vi "MultiClassTable.vi"() -> ()   [LabVIEW 2013]
uses:
  ColumnVIs/Column/Column.lvclass
  ColumnVIs/ModeCol/ModeCol.lvclass
  ColumnVIs/GroupCol/GroupCol.lvclass
  ColumnVIs/DigitalCol/DigitalCol.lvclass
  ColumnVIs/TriggerCol/TriggerCol.lvclass
  ColumnVIs/SingleValCol/SingleValCol.lvclass
  <vilib>/event_ctls.llb/eventvkey.ctl
  <vilib>/Utility/miscctls.llb/LVRowAndColumnTypeDef.ctl
  TypeDefs/RowType.ctl
  TypeDefs/TableHistory.ctl
  TypeDefs/TableArray.ctl
  TypeDefs/AddDeviceRing.ctl
  DeviceVIs/Device/Device.lvclass
  TypeDefs/PreviousVersionSelect.ctl
  VariableManagerCodes/VariableManager/VariableManager.lvclass
  <vilib>/Utility/miscctls.llb/LVRowAndColumnUnsignedTypeDef.ctl
  PackedLibraries/LuaEvaluatorAPI.lvlibp/API/t_Caching_Expression_Evaluator_Methods_v4.ctl
  TypeDefs/ClickEvent.ctl
  <vilib>/Utility/miscctls.llb/LVPoint32TypeDef.ctl
  <vilib>/Utility/error.llb/DialogType.ctl
  TypeDefs/SaveCluster.ctl
  <vilib>/Utility/miscctls.llb/LVStringsAndValuesArrayTypeDef_I32.ctl
  <vilib>/Utility/cursorutil.llb/Set Cursor (Icon Pict).vi
  DeviceVIs/NextMaster_v4.vi
  PackedLibraries/LuaEvaluatorAPI.lvlibp
  DeviceVIs/SubVIs.lvlib
  VariableManagerCodes/API/VariableManagerAPI.lvlib
panel:
  out "Button\n(Mouse Down?)":u16
  out "Index Values":T1
  out "Igor Inform Array":string[](array[string])
  out "Devices queue":refnum<queue>
  in  "UpdateHWI Button":bool
  in  "StopExperiment":bool
  in  "Run Seq Button":bool
  in  "Run Button":bool
  in  "Cycle":bool
  in  "RandomSequence":bool
  in  "VariableManager":refnum<class "VariableManager.lvclass">=refnum
  out "CycleX Event":refnum<user-event>
  out "Dyn.\nRegist.\nCycleX\nEvent":refnum<event-registration>
  out "Dyn.\nRegist.\nSeq.\nEvent":refnum<event-registration>
  out "Dyn. Regist. Update Event":refnum<event-registration>
  out "Update Notifier":refnum<notifier>
  out "Update Event":refnum<user-event>
  out "Seq. Event":refnum<user-event>
  out "Loaded Version":string="testing"
  out "Procedure Name":string="test_branch"
  in  "Tab Control":T2(tab)=enum."Variables"
  in  "Program only changes":bool=TRUE
  out "SequenceHistory":string[][](table)
  in  "File Number":i32
  in  "Program during MOT loading":bool
  in  "Additional wait time (s)":dbl
  out "Igor Inform String":string
  in  "FitCol2Text Button":bool
  in  "SetList Table":string[][](table)=[["initialize", "", "Ramp", "1", "1", "0", "0", "0", "0", "0", "0", "0", "0", "0", "0", "0", "0", "0", "0", "0", "0", "0", "0", "0", "0", "0", "0", "0", "0", "100m"]]
  in  "Undo":bool
  in  "Redo":bool
  in  "Select Layout":i32(ring)=-1 items=["(On-the-fly)"=-2, "All"=-1]
  in  "ConfigLayoutsButton":bool
  in  "Add Device":T3 items=["Select Type...", "DDS", "Novatech", "NI Card"]
  in  "ManageDevicesButton":bool
  in  "User defined functions":string="-- --------------------------------------------------------------------------\n-- RbYb Beatnote Command \"frequency\" functions\n--      These functions allow us to run a sequence using absolute frequency \n--      detuning by calculating the proper command \"frequency\"\n--\n--      NOTE: Only use one TA or Re \"comm\" function, or it isn't clear which setpoint will be used\n--\n--      18.Aug.2010: Updated Master AOM offset (40 --> 42.342).\n-----------------------------------------------------------------------------\nfunction TASlowComm(Detuning,AOM)\n    return (-1*Detuning+1126.48-60.32-42.342-2*AOM)/8\n   --positive detuning is BLUE detuned, zero detuning sets TA slower beam to the 87-Rb F=2 to F'=3\nend\n\nfunction TAMOTComm(Detuning,AOM)\n    return (-1*Detuning+1126.48-60.32-42.342+AOM)/8\n   --positive detuning is BLUE detuned, zero detuning sets TA MOT beam to the 87-Rb F=2 to F'=3\nend\n\nfunction TAPComm(Detuning,AOM)\n    return (-1*Detuning+1126.48-60.32-42.342+AOM)/8\n   --positive detuning is BLUE detuned, zero detuning sets TA Probe beam to the 87-Rb F=2 to F'=3\nend\n\nfunction ReMOTComm(Detuning,AOM)\n    return (Detuning+6568.03-1126.48+60.32+42.342-2*AOM)/64\n    --positive detuning is BLUE detuned, zero detuning sets Repump MOT beam to the 87-Rb F=1 to F'=2\nend\n\nfunction ReSlowComm(Detuning,AOM)\n    return (Detuning+6568.03-1126.48+60.32+42.342+2*AOM)/64\n    --positive detuning is BLUE detuned, zero detuning sets Repump slower beam to the 87-Rb F=1 to F'=2\nend\n\n--RbLi Probe (transverse coolign launch)\nfunction PComm(Detuning)\n    return (-1*Detuning+986.16)/8\n    --positive detuning is BLUE detuned, zero detuning sets Repump slower beam to the 87-Rb F=1 to F'=2\nend\n\n-- Creates an exponential ramp from A to B in tEnd seconds\n-- useful for stopping a ramp at different times to measure T, N\nfunction ExpRampStep(t, a, b, tau, tEnd)\n   return (b - a*exp(tEnd / tau) + (a-b)*exp(t/tau))/ ( 1 - exp(tEnd / tau) );\nend\n\nfunction ExpRampEnd(tEv, a, b, tau, tEnd)\n   return (b - a*exp(tEnd / tau) + (a-b)*exp(tEv/tau))/ ( 1 - exp(tEnd / tau) );\nend\n\nfunction ExpRamp2(t,a,tau)\n   return a*exp(-t/tau)\nend\n\nfunction ExpRamp2End(tEnd,a,tau)\n   return a*exp(-tEnd/tau)\nend\n\n-- Added log chip amplifier (1 V per decade) so now we provide linear ramp to get exponential\n--     note: log() is base 'e', log10 base '10'\nfunction LineEvap(t,a,tau)\n   return 1.027*(log10(a)-t/(2.30*tau))+0.0343\nend\n\n-- final value log(V) for LineEvap\nfunction LineEvapEnd(tEnd,a,tau)\n   return 1.027*(log10(a)-tEnd/(2.30*tau))+0.0343\nend\n\n-- Convert real dipole power to log chip request V\nfunction PtoV(pow)\n   return 1.010*log10(pow/0.770)\nend\n\n-- Convert 532 horizontal (main) beam power (in mW) to V-req\nfunction PtoV532m(pow)\n   return 1.01378*log10(pow/0.54672)\nend\n\n-- Convert 532 vertical (crossing) beam power (in mW) to V-req\nfunction PtoV532c(pow)\n   return 1.03459*log10(pow/0.619665)\nend\n\n-- Convert 1064 horizontal (main) beam power (in mW) to V-req\nfunction PtoV1064m(pow)\n   return 1.0035*log10(pow/1.2104)\nend\n----------------------------------------\n-- The following functions are part of the \"standard load\" of functions and should not be messed with\n-- They are here for reference only.\n-- Please add any user functions above this comment\n-- -------------------------------------------------------------------------------------------\n\n-- Creates a linear ramp from A to B\nfunction LineRamp(f, Initial, Final)\n    return (1-f)*Initial + f*Final;\nend\n\n-- Creates an exponential ramp from A to B\nfunction ExpRamp(t, a, b, tau)\n   return (b - a*exp(tMax / tau) + (a-b)*exp(t/tau))/ ( 1 - exp(tMax / tau) );\nend\n\n-- Creates a sinewave\nfunction SinRamp(t,Offset,A,Freq, Phase)\n    return Offset + A * sin(2*pi*Freq*t + Phase)\nend\n\n-- Creates a blackman pulse\nfunction Blackman(f, Offset, A)\n    return Offset +  A*sqrt(0.5*cos(3.1415*(2*f-1))+0.08*cos(2*pi*(2*f-1))+0.42);\nend\n\n-- Creates a half-gauss ramp\nfunction HalfGaussRamp(t, a, b, Width)\n    local y;\n    y = exp(-(tMax^2)/Width^2);\n    y = (a -  b*y)/(1-y)  +  ((b-a)/(1-y))*exp(-((t-tMax)^2)/Width^2);\n    return y;\nend\n\n-- Creates an \"O'Hara\" ramp from A to B, for dipole evaporation\nfunction EvapRamp(t, a, b, tau)\n   local y;\n  y = log(a/b) / log(1+tMax/tau);\n  y = a * (1+t/tau)^(-y);\n  return y;\nend\n"
  out "Loading Text":string="Loading..."
  in  "Version Selection":T4=enum."Load DDS 4.10"
  in  "Old HWGlobals Path":path=path "C:/Experiment/Data Acquisition/Hardware Control/Hardware/2014/6Jun2014_PowerCal" caption="This file has not been loaded or saved"
  in  "Old HWGlobals History":string(combo)
  in  "Old Procedure Path":path=path "C:/Experiment/Data Acquisition/Hardware Control/procedures/Benchmarks/12Feb2014_RbQuad" caption="This file has not been loaded or saved"
  in  "Old Procedure History":string(combo)
  in  "Load Old":bool
  in  "Load Recent":string(combo)
  in  "Save to Disk":bool
  in  "Load from Disk":bool
  out "Table error":errorcluster
  out "Sequencing Error":errorcluster
  out "Update Error":errorcluster
  in  "Debug: apply appearance":bool
  out "DevNums":i32[](array[numeric])=[0, 0, 0, 0, 0, 0, 0, 0, 0, 0, 0, 0, 0, 0, 0, 0, 0, 0, 0, 0, 0, 0, 0, 0, 0, 0, 0, 0, 0, 0, 1, 1, 1, 1, 1, 1, 1, 1, 1, 1, 1, 1, 1, 1, 1, 1, 1, 1, 1, 1, 2, 2, 2, 2, 2, 2, 2, 2, 2, 2, 2, 2, 2, 2, 2, 2, 2, 2, 2, 2, 3, 3, 3, 3, 3, 3, 3, 3, 3, 3, 3, 3, 3, 3, 3, 3, 3, 3, 3, 3, 4, 4, 4, 4, 4, 4, 4, 4, 5, 5, 5, 5, 5, 5, 5, 5, 5, 5, 5, 5, 6, 6, 6, 6, 6, 6, 6, 6, 6, 6, 6, 6, 7, 7, 7, 7, 7, 7, 7, 7, 7, 7, 7, 7]
  in  "Devices":refnum<class "Device.lvclass">[](array[class])
  in  "PreserveHist?":bool
  out "Hist. size":i32=2
  out "#chg":i16
  out "Defer Pnl Upd":bool=TRUE
  out "diag. loop cnt":i32
  out "Key Focus":bool
  out "Edit Position":T5={"Row"=-2, "Column"=-2}
  out "withinSelection?":bool
  out "Val Change":bool=TRUE
  out "Selection Size":T5
  in  "row type":T6=enum."within data"
  out "Selection Start":T5={"Row"=25, "Column"=30}
  out "Char":i16
  out "VKey":T7
  out "withinData?":bool=TRUE
  out "data cols":i32=134
  out "data rows":i32=26
  out "Number of Rows":u32=36
  out "Number of Columns":u32=62
  out "Table History":T8
  in  "Diag. loop?":bool
  in  "Defer Updates?":bool=TRUE
  out "Clipboard":string[][](array[string])
  out "Col array":refnum<class "Column.lvclass">[](array[class])
  in  "quit":bool
  in  "initialize?":bool
  # "Use the quit button -->\nPressing stop causes problems with Variable Manager"
  # "(must abort to stop,\nstill better to QUIT first)"
  # "diagnostics:"
  # "presently not set\nfor row header"
  # "The table size in (rows, cols) is NOT same as\nthe size of the data array displayed in table."
  # "Necessary table settings:\n - Show column/row headers (Properties)\n - No editable headers (unless we'll handle all column header clicks)"
  # "\"Diagnostics\" we can't delete:\nRow Type, ..."
  # "What do we actually need from old CycleX here?\n   - Inform Igor?\n   - Program changes/ during MOT load?"
  # "(not presently implemented)"
  # "Sequencing controls to add: Run Sequence/Abort, Sequence Step indicator, Randomize?, Mulligans"
  # "Variable Manager will be initialized when the VI is run.\n\nIf it is currently running and you can see this message, then you've \"popped out\" the Variable manager.\nClose it with the \"red-x\" to replace it here."
  # "Note: For each index <idx>, the names <idx>_f and <idx>_max\nare also defined as the fractional sequence step and max steps."
  # "In the context of ramps several variables are passed or specified that may be used here:\n\n   - f the fractional position of a point in a ramp\n   - t the current time in a ramp\ndt the current timestep size.\ntMax the total duration of the ramp\n\ntemporary \"storage\":\n-- not functionality for strings (always treated as double)\nfunction bnot(a)\n   -- this \"(bool exp.) and b or c\" is equivalent to \"(bool exp.) ? b : c\" syntax.\n   -- caution: undefined variables evaluate to \"false\" so will NOT throw an error as argument\n   return a==0 and 1 or 0\nend"
  # "Present Version"
  # "Save/Load from present version (select single file):\nWe need to save the following:\n   - Devices (with the columns and data pushed from table first!)\n   - Layout ring (for layout names, #s)\n   - variables\n   - user functions\n   - ... ?"
  # "Load... and Save... bring up dialog box.\nLoad Recent will load the selected procedure. BUG: not a value change if select what's on top!"
  # "Previous Versions"
  # "Load from older versions (select Procedure and Hardware globals)\n(1) reformat old file to give device array\n(2) collect variables and send them to variable manager\n(3) load user functions\n(4) construct layouts, if any (at least a default \"all on\" layout)\n(5) ...?"
  # "Notes:\n\nVariables used in digital columns are interpreted as high for any value not equal to 0, and low for 0."
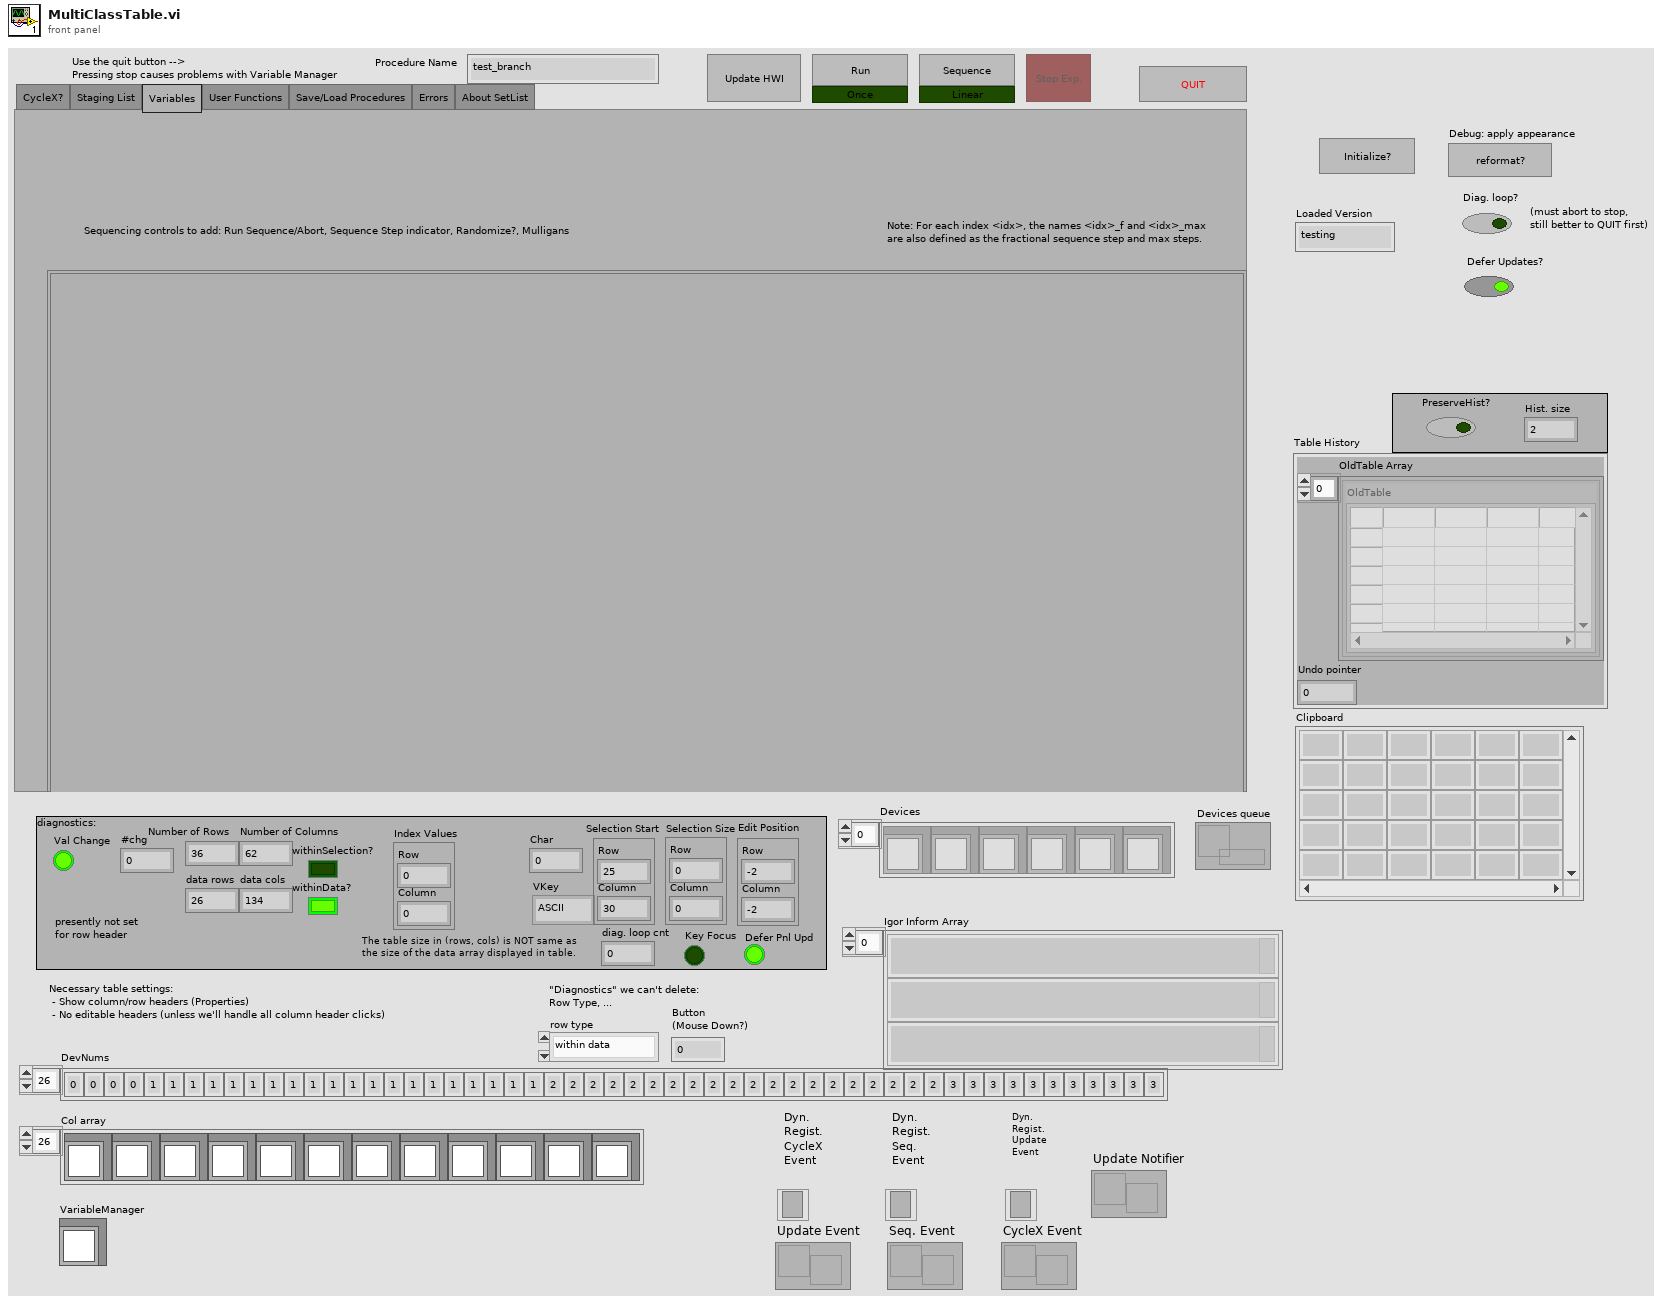
[diagram p1: front panel]
types:
  T1 = typedef "LVRowAndColumnUnsignedTypeDef.ctl" = cluster{"Row":u32, "Column":u32}
  T2 = enum32{"CycleX?", "Staging List", "Variables", "User Functions", "Save/Load Procedures", "Errors", "About SetList"}
  T3 = typedef "AddDeviceRing.ctl" = u16
  T4 = typedef "PreviousVersionSelect.ctl" = enum32{"Load PreDDS 4.10", "Load early 2009 files", "Load 2009-2010 files", "Load DDS 4.10", "Load v4.09"}
  T5 = typedef "LVRowAndColumnTypeDef.ctl" = cluster{"Row":i32, "Column":i32}
  T6 = typedef "RowType.ctl" = enum16{"below data", "within data", "column header", "first row"}
  T7 = typedef "eventvkey.ctl" = enum16{"ASCII", "Enter", "Return", "Shift", "Ctrl", "Alt", "Cmd", "Opt", "Caps", "NumLock", "Clear", "Break", "Up", "Down", "Left", "Right", "Insert", "Delete", "Home", "End", "PageUp", "PageDown", "Escape", "Help", "Pause", "ScrollLock", "F1", "F2", "F3", "F4", "F5", "F6", "F7", "F8", "F9", "F10", "F11", "F12", "F13", "F14", "F15", "F16", "F17", "F18", "F19", "F20", "F21", "F22", "F23", "F24", "Play", "VolumeUp", "VolumeDown", "Mute", "Two Byte Char"}
  T8 = typedef "TableHistory.ctl" = cluster{"OldTable Array":T9, "Undo pointer":i32}
  T9 = typedef "TableArray.ctl" = cluster{"OldTable":string[][]}[]
  T10 = enum8{"Enabled", "Disabled", "Disabled and Grayed Out"}
  T11 = typedef "LuaEvaluatorAPI.lvlibp/t_Caching_Expression_Evaluator_Methods_v4.ctl" = enum16{"set", "get", "eval", "eval2", "assign", "execute", "isvalid"}
  T12 = typedef "ClickEvent.ctl" = cluster{"CtlRef":refnum<vi>, "Coords":T13, "Button":u16, "Mods":cluster{"Double Click":bool, "Menu Key":bool}, "PlatMods":cluster{"Shift":bool, "Ctrl":bool, "Alt":bool, "Cmd":bool, "Opt":bool}}
  T13 = typedef "LVPoint32TypeDef.ctl" = cluster{"Horizontal":i32, "Vertical":i32}
  T14 = typedef "SaveCluster.ctl" = cluster{"Version":string, "Devices":refnum<class "Device.lvclass">[], "Select Layout":i32, "Layout:Strings And Values []":T15, "User defined functions":string, "VariableManager":refnum<class "VariableManager.lvclass">}
  T15 = typedef "LVStringsAndValuesArrayTypeDef_I32.ctl" = cluster{"String":string, "Value":i32}[]
  T16 = cluster{"Shift":bool, "Ctrl":bool, "Alt":bool, "Cmd":bool, "Opt":bool}
  T17 = typedef "ClickReturn.ctl" = cluster{"Button":u16, "Mods":cluster{"Double Click":bool, "Menu Key":bool}, "PlatMods":cluster{"Shift":bool, "Ctrl":bool, "Alt":bool, "Cmd":bool, "Opt":bool}, "Discard?":bool}
  T18 = typedef "DialogType.ctl" = u16
  T19 = typedef "ColumnLayoutCluster.ctl" = cluster{"Label":string, "Color":u32, "Width":u32, "[disp?]":bool[]}
  T20 = cluster{"left":i16, "top":i16, "right":i16, "bottom":i16}
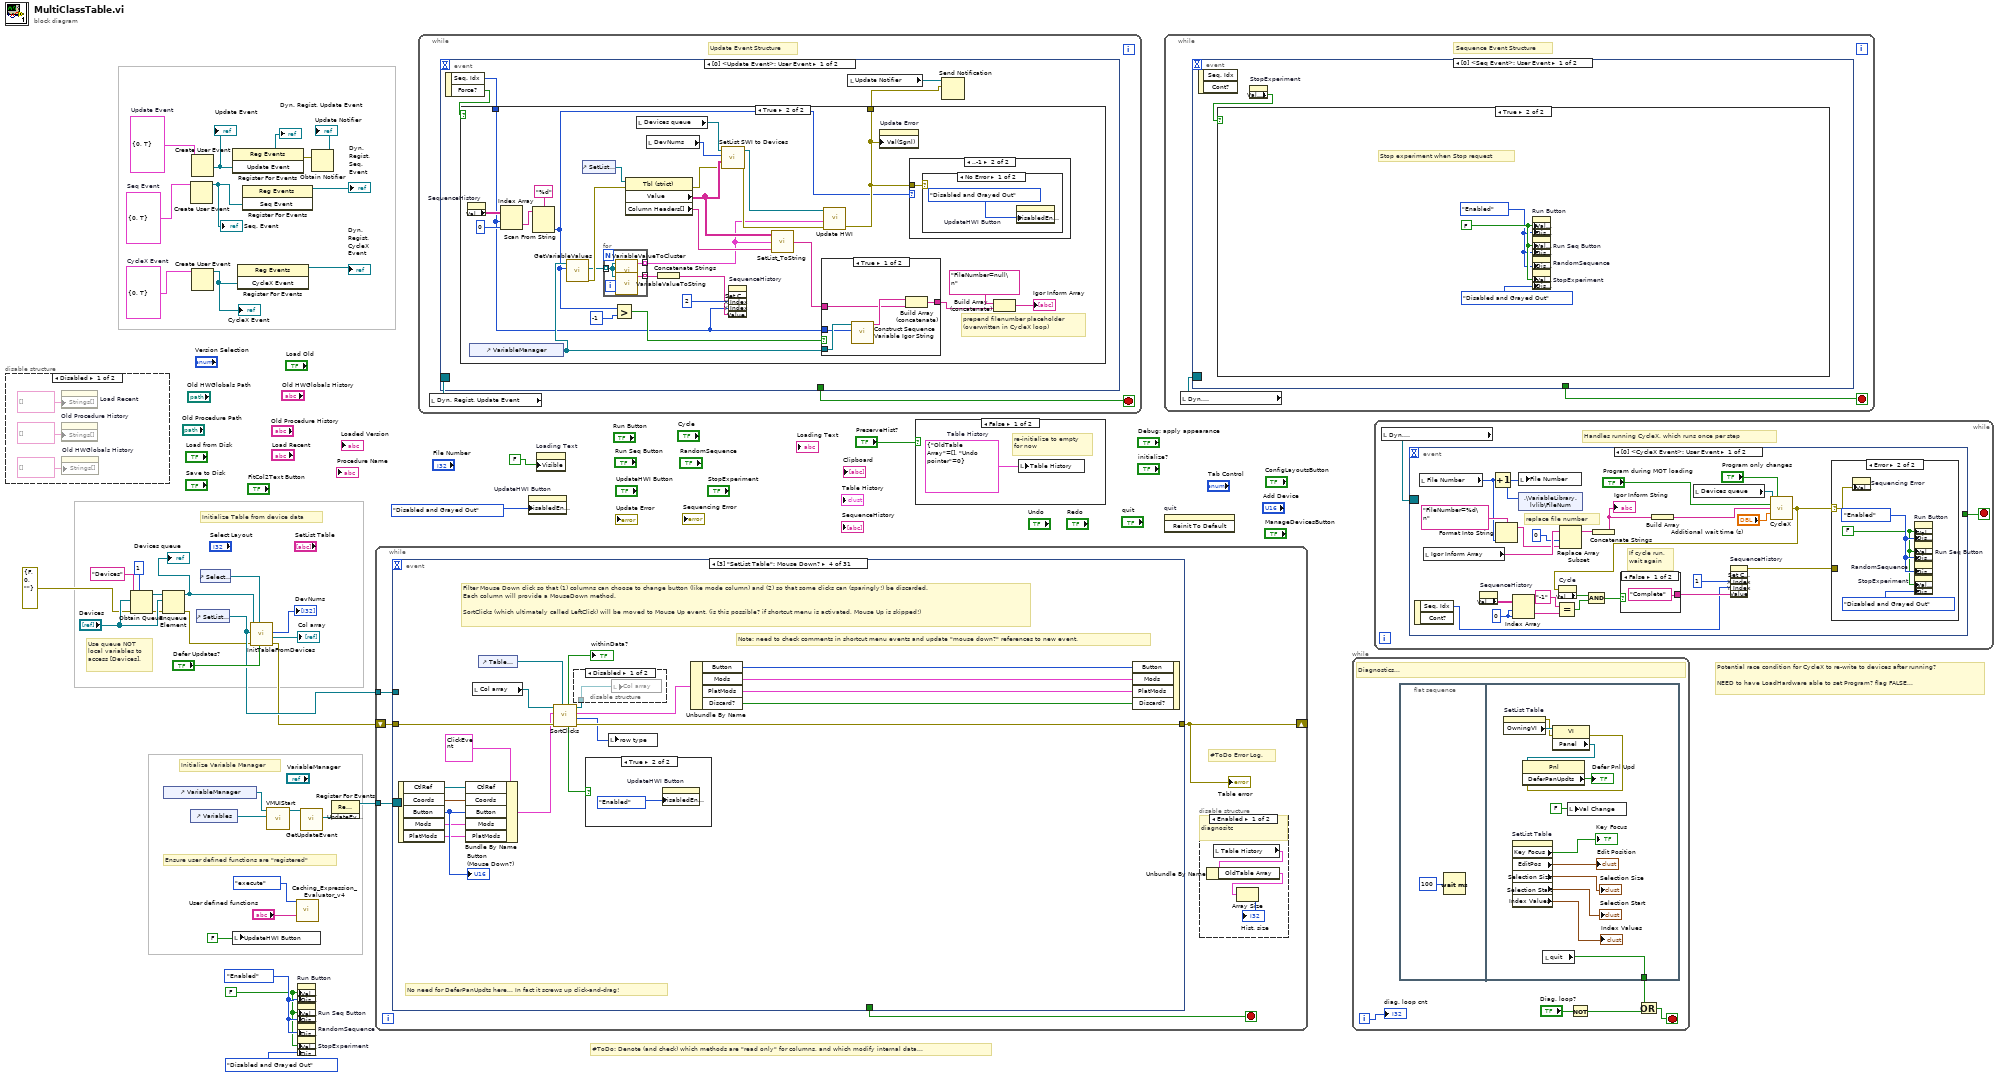
[diagram p0: block diagram]
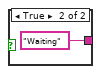
[diagram p2: hidden frame]
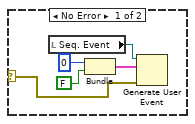
[diagram p3: hidden frame]
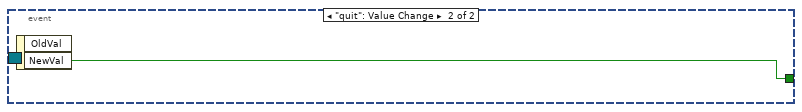
[diagram p4: hidden frame]
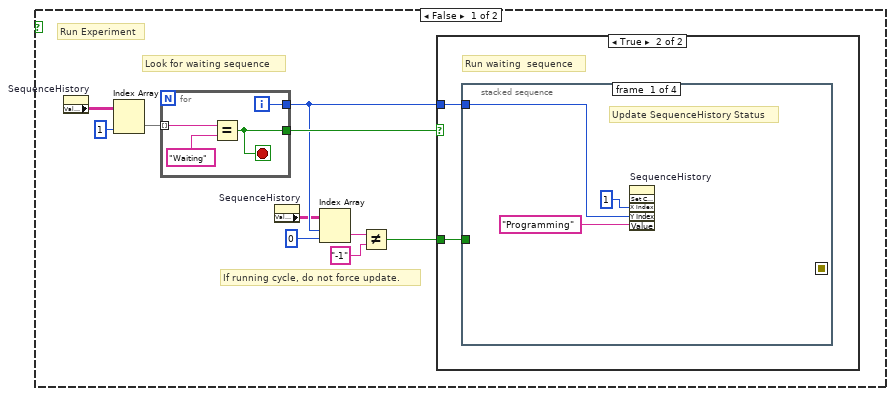
[diagram p6: hidden frame]
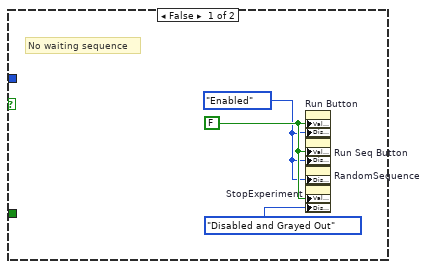
[diagram p7: hidden frame]
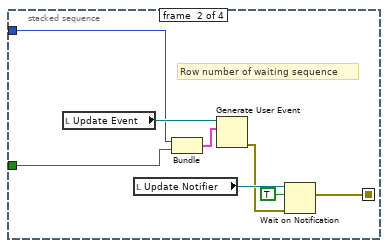
[diagram p8: hidden frame]
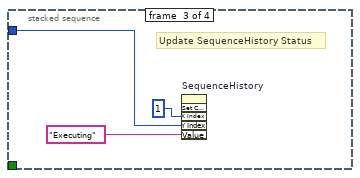
[diagram p9: hidden frame]
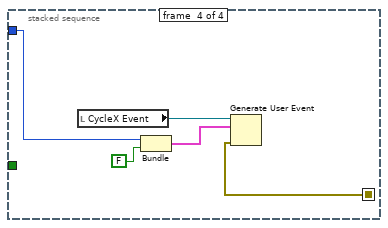
[diagram p10: hidden frame]
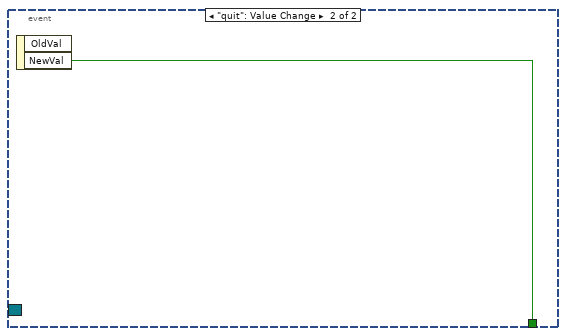
[diagram p11: hidden frame]
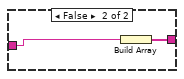
[diagram p15: hidden frame]
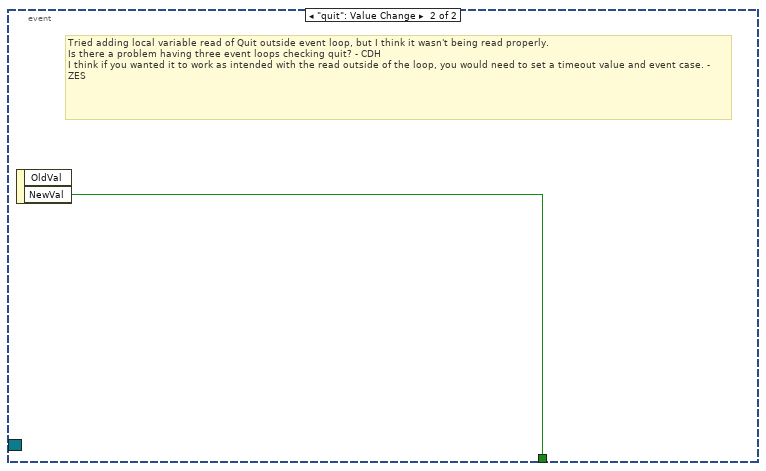
[diagram p16: hidden frame]
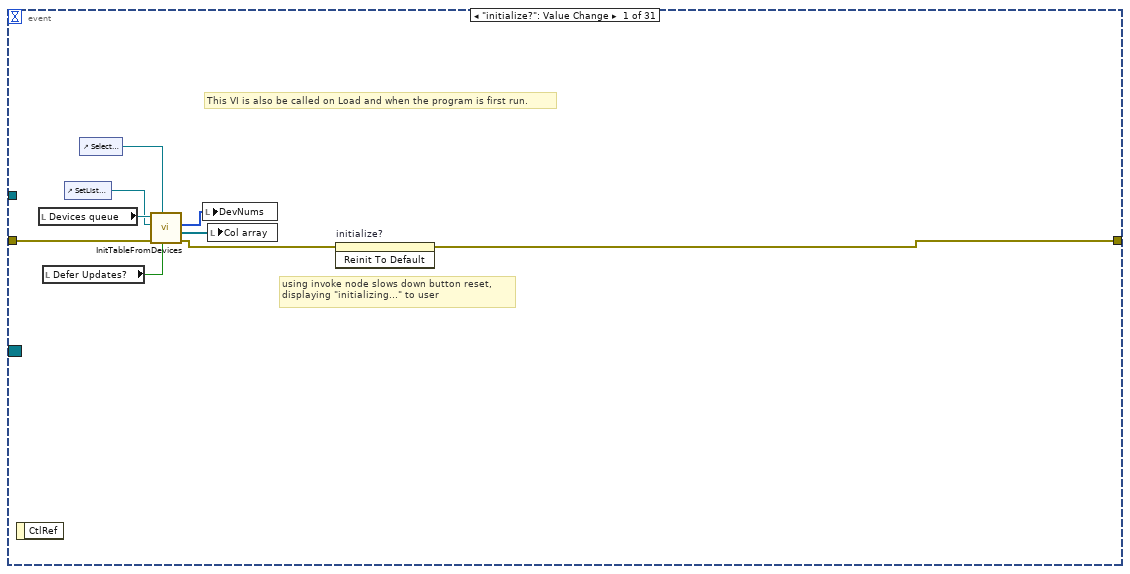
[diagram p19: hidden frame]
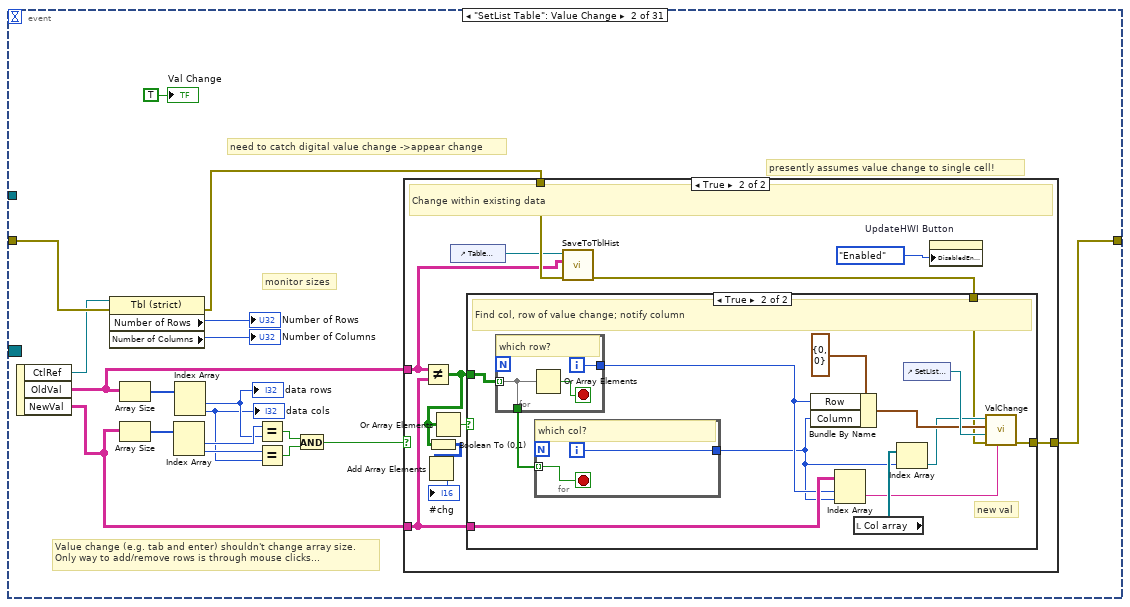
[diagram p20: hidden frame]
diagram:
  w13 = T10."Enabled" ("Disabled")
  w12 = FALSE
  w24 = cluster{"Seq. Idx":i32, "Cont?":bool} {"Seq. Idx"=0, "Cont?"=TRUE}  # CycleX Event
  w36 = cluster{"Seq. Idx":i32, "Cont?":bool} {"Seq. Idx"=0, "Cont?"=TRUE}  # Seq Event
  w37 = cluster{"Seq. Idx":i32, "Force?":bool} {"Seq. Idx"=0, "Force?"=TRUE}  # Update Event
  # "Use queue NOT\nlocal variables to\naccess [Devices]."
  # "Potential race condition for CycleX to re-write to devices after running?\n\nNEED to have LoadHardware able to set Program? flag FALSE..."
  # "Ensure user defined functions are \"registered\""
  # "Initialize Variable Manager"
  # "Initialize Table from device data"
  # "#ToDo: Denote (and check) which methods are \"read only\" for columns, and which modify internal data..."
  n1 = disable-structure shown="Disabled" {
    frame Disabled {
      n2 = property on="Load Recent" class="CmbBox"("Strings[]"=string[] [] ("Strings []")) -> ()  [unwired: 2 in, 2 out]
      n3 = property on="Old Procedure History" class="CmbBox"("Strings[]"=string[] [] ("Strings []")) -> ()  [unwired: 2 in, 2 out]
      n4 = property on="Old HWGlobals History" class="CmbBox"("Strings[]"=string[] [] ("Strings []")) -> ()  [unwired: 2 in, 2 out]
    }
    frame Enabled {
    }
  }
  n5 = Obtain Queue(max queue size (-1, unlimited)=1, name (unnamed)="Devices", element data type="Devices", error in (no error)=errorcluster {"status"=FALSE, "code"=0, "source"=""} ("error out")) -> (queue out=w5:refnum<queue>, error out=w4:errorcluster)  [unwired: 1 in, 1 out]
  n6 = Enqueue Element(queue=w5, element="Devices", error in (no error)=w4) -> (queue out=w1:refnum<queue>, error out=w3:errorcluster)  [unwired: 1 in, 1 out]
  "Devices queue" <- w1
  n7 = control-ref of="VariableManager"() -> (w16:refnum<vi>)
  n8 = control-ref of="Variables"() -> (w15:refnum<vi>)
  n9 = Create User Event(user event datatype=w36) -> (user event=w21:refnum<user-event>)  [unwired: 1 in, 1 out]
  "Seq. Event" <- w21
  n10 = Create User Event(user event datatype=w37) -> (user event=w38:refnum<user-event>)  [unwired: 1 in, 1 out]
  "Update Event" <- w38
  n11 = Create User Event(user event datatype=w24) -> (user event=w23:refnum<user-event>)  [unwired: 1 in, 1 out]
  "CycleX Event" <- w23
  n12 = control-ref of="SetList Table"() -> (w18:refnum<vi>)
  n13 = control-ref of="Select Layout"() -> (w30:refnum<vi>)
  n14 = register-events(w38) -> (reference out=→"Dyn. Regist. Update Event":refnum<event-registration>, error out=w32:errorcluster)  [unwired: 2 in]
  n15 = local write "UpdateHWI Button"(FALSE ("UpdateHWI Button")) -> ()
  n16 = register-events(w23) -> (reference out=→"Dyn.\nRegist.\nCycleX\nEvent":refnum<event-registration>)  [unwired: 2 in, 1 out]
  n17 = register-events(w21) -> (reference out=→"Dyn.\nRegist.\nSeq.\nEvent":refnum<event-registration>)  [unwired: 2 in, 1 out]
  n18 = call "InitTableFromDevices.vi"("Defer Updates? (T)"="Defer Updates?", "Layout Ref"=w30, "error in (no error)"=w3, "Table Ref in"=w18, "Devices queue"=w1) -> ("error out"=w17:errorcluster, "Col array"=→"Col array":refnum<class "Column.lvclass">[], "DevNums"=→"DevNums":i32[])  [unwired: 3 in, 1 out]
  n19 = call "VMUIStart.vi"("SubPanelRef"=w15, "VariableManagerRef in"=w16) -> ("VariableManagerRef out"=w11:refnum<vi>)  [unwired: 8 in, 1 out]
  n20 = call "Caching_Expression_Evaluator_v4.vi"("method"=t_Caching_Expression_Evaluator_Methods_v4."execute", "expression/scriptlet"="User defined functions") -> ()  [unwired: 12 in, 2 out]
  n21 = property on="Run Button" class="Bool (strict)"("Value"=w12, "DisabledEnum"=w13) -> ()  [unwired: 2 in, 2 out]
  n22 = property on="Run Seq Button" class="Bool (strict)"("Value"=w12, "DisabledEnum"=w13) -> ()  [unwired: 2 in, 2 out]
  n23 = property on="RandomSequence" class="Bool (strict)"("DisabledEnum"=w13) -> ()  [unwired: 2 in, 2 out]
  n24 = property on="StopExperiment" class="Bool (strict)"("Value"=w12, "DisabledEnum"=T10."Disabled and Grayed Out" ("Disabled")) -> ()  [unwired: 2 in, 2 out]
  n25 = call "GetUpdateEvent.vi"("VariableManagerRef in"=w11) -> ("UpdateEvent"=w10:refnum<user-event>)  [unwired: 8 in, 2 out]
  n26 = Obtain Notifier(notification data type=w32) -> (notifier out=→"Update Notifier":refnum<notifier>)  [unwired: 3 in, 2 out]
  n27 = register-events(w10) -> (reference out=w9:refnum<event-registration>)  [unwired: 2 in, 1 out]
  n28 = while {
    shift-right: [w45] -> _
    shift-left: w17 -> [w46]
    tunnel: w18 -> [w44]
    tunnel: w9 -> [w43]
    stop <- w47 stop-if-true
    # "#ToDo Error Log."
    n29 = event shown="[3] \"SetList Table\": Mouse Down?" {
      selector: w43 -> [_ _ _ _ _ _ _ _ _ _ _ _ _ _ _ _ _ _ _ _ _ _ _ _ _ _ _ _ _ _ _]
      dyn-events: _ -> [_ _ _ _ _ _ _ _ _ _ _ _ _ _ _ _ _ _ _ _ _ _ _ _ _ _ _ _ _ _ _]
      timeout: _ -> [_ _ _ _ _ _ _ _ _ _ _ _ _ _ _ _ _ _ _ _ _ _ _ _ _ _ _ _ _ _ _]
      tunnel: [_ _ _ _ _ _ _ _ _ _ _ _ _ _ _ w477 _ _ _ _ _ _ _ _ _ _ _ _ _ _ _] -> w47
      tunnel: [w51 w61 w115 w215 _ w281 w298 w316 w319 w324 w341 w350 w365 w431 _ w468 w484 w510 _ _ _ _ _ _ w639 _ _ w652 _ _ _] -> w45
      tunnel: w46 -> [w54 w65 w114 w216 w231 w280 w310 w317 w320 w325 w344 w352 w368 w428 _ w471 w482 w512 _ _ _ _ _ _ w635 _ _ _ _ _ _]
      tunnel: w44 -> [_ _ _ _ _ _ _ _ _ _ w340 _ w367 w426 _ _ w480 w507 _ _ _ _ _ _ _ _ _ _ _ _ _]
      event "initialize?": Value Change {
        # "using invoke node slows down button reset,\ndisplaying \"initializing...\" to user"
        # "This VI is also be called on Load and when the program is first run."
        n30 = event-data() -> ()  [unwired: 1 in, 1 out]
        n31 = local read "Devices queue"() -> (w59:refnum<queue>)
        n32 = local read "Defer Updates?"() -> (w53:bool)
        n33 = control-ref of="SetList Table"() -> (w56:refnum<vi>)
        n34 = control-ref of="Select Layout"() -> (w55:refnum<vi>)
        n35 = call "InitTableFromDevices.vi"("Defer Updates? (T)"=w53, "Layout Ref"=w55, "error in (no error)"=w54, "Table Ref in"=w56, "Devices queue"=w59) -> ("error out"=w52:errorcluster, "Col array"=w57:refnum<class "Column.lvclass">[], "DevNums"=w58:i32[])  [unwired: 3 in, 1 out]
        n36 = local write "DevNums"(w58) -> ()
        n37 = local write "Col array"(w57) -> ()
        n38 = invoke on="initialize?" class="Bool (strict)" method="Reinit To Default"(error in=w52) -> (error out=w51:errorcluster)  [unwired: 2 in, 2 out]
      }
      event "SetList Table": Value Change {
        # "presently assumes value change to single cell!"
        # "need to catch digital value change ->appear change"
        # "Value change (e.g. tab and enter) shouldn't change array size.\nOnly way to add/remove rows is through mouse clicks..."
        # "monitor sizes"
        n39 = event-data() -> ("CtlRef"=w64:refnum<vi>, "OldVal"=w66:string[][], "NewVal"=w63:string[][])  [unwired: 1 in]
        n40 = property on="Property Node" class="Tbl (strict)"(reference=w64, error in=w65) -> (error out=w62:errorcluster, "Number of Rows"=→"Number of Rows":u32, "Number of Columns"=→"Number of Columns":u32)  [unwired: 1 out]
        n41 = Array Size(array=w66) -> (size(s)=w74:i32[])
        n42 = Array Size(array=w63) -> (size(s)=w77:i32[])
        n43 = Index Array(array=w77) -> (element #1=w73:i32, element #2=w72:i32)  [unwired: 2 in]
        n44 = Index Array(array=w74) -> (element #1=w69:i32, element #2=w68:i32)  [unwired: 2 in]
        "data rows" <- w69
        "data cols" <- w68
        n45 = Equal?(x=w73, y=w69) -> (x = y?=w70:bool)
        n46 = Equal?(x=w72, y=w68) -> (x = y?=w71:bool)
        n47 = And(x=w70, y=w71) -> (x .and. y?=w67:bool)
        n48 = case shown="True" w67 {
          tunnel: w66 -> [w79 w85]
          tunnel: w63 -> [_ w89]
          tunnel: w62 -> [w78 w86]
          tunnel: [w78 w90] -> w61
          frame False {
            # "non-allowed resize:\nrevert back to previous table"
            # "Changed outside existing data; discard"
            n49 = local write "SetList Table"(w79) -> ()
          }
          frame True {
            # "Change within existing data"
            n50 = Not Equal?(x=w85, y=w89) -> (x != y?=w83:bool[][])
            n51 = Boolean To (0,1)(Boolean=w83) -> (0, 1=w82:i16[][])
            n52 = Add Array Elements(numeric array=w82) -> (sum=→"#chg":i16)
            n53 = Or Array Elements(Boolean array=w83) -> (logical OR=w88:bool)
            n54 = control-ref of="Table History"() -> (w84:refnum<vi>)
            n55 = call "SaveToTblHist.vi"("error in (no error)"=w86, "OldTable (reset)"=w85, "Table History ref"=w84) -> ("error out"=w87:errorcluster)  [unwired: 8 in]
            n56 = case shown="True" w88 {
              tunnel: w83 -> [_ w104]
              tunnel: w87 -> [w91 w92]
              tunnel: [w91 w100] -> w90
              tunnel: w89 -> [_ w96]
              frame False {
                # "No value change! (debugging event)"
              }
              frame True {
                # "new val"
                # "Find col, row of value change; notify column"
                n57 = for {
                  tunnel: w104 -> [w108] mode=indexing
                  tunnel: [w108] -> w103
                  tunnel: [w107] -> w95
                  i -> [w107]
                  stop <- w109 stop-if-true
                  # "which row?"
                  n58 = Or Array Elements(Boolean array=w108) -> (logical OR=w109:bool)
                }
                n59 = for {
                  tunnel: w103 -> [w105] mode=indexing
                  tunnel: [w106] -> w94
                  i -> [w106]
                  stop <- w105 stop-if-true
                  # "which col?"
                }
                n60 = Bundle By Name(cluster=T5 {"Row"=0, "Column"=0} ("Cell Position"), "Row"=w95, "Column"=w94) -> (w98:T5)
                n61 = Index Array(array=w96, index (row)=w95, index (col)=w94) -> (element=w93:string)
                n62 = local read "Col array"() -> (w101:refnum<class "Column.lvclass">[])
                n63 = Index Array(array=w101, index=w94) -> (element=w97:refnum<class "Column.lvclass">)
                n64 = control-ref of="SetList Table"() -> (w99:refnum<vi>)
                n65 = call-dynamic "ValChange.vi"("Value"=w93, "error in (no error)"=w92, "Table CtlRef In"=w99, "Cell Position"=w98, "Column in"=w97) -> ("error out"=w100:errorcluster)  [unwired: 4 in, 2 out]
              }
            }
            n66 = property on="UpdateHWI Button" class="Bool (strict)"("DisabledEnum"=T10."Enabled" ("Disabled")) -> ()  [unwired: 2 in, 2 out]
          }
        }
        "Val Change" <- TRUE ("Val Change")
      }
      event "SetList Table": Key Down? {
        # "#ToDo: Copy/Paste not working... \nAccording to the LabVIEW help files, Ctrl-V or any menu-shortcut CANNOT be repurposed,\neven if the menus are hidden!"
        # "Selection start is initially placed at the edit on mouse press, so it provides (row, col). However keyboard motion (default Return, Tab behavior) doesn't move it.\nTo re-enable keyboard navigation (and to add arrow keys), one needs to force selection start to move so it can be checked on each key stroke!\n\nRevisit this: After mouse handling \"paradigm\" has been re-worked, this should be easier to include. See Sandbox/TableSanbox.vi (Key Down event) for ideas."
        n67 = event-data() -> ("CtlRef"=w118:refnum<vi>, "Char"=w122:i16, "VKey"=w121:T7, "PlatMods"=w120:T16)  [unwired: 1 in, 3 out]
        "VKey" <- w121
        "Char" <- w122
        n68 = local read "Devices queue"() -> (w110:refnum<queue>)
        n69 = control-ref of="Table History"() -> (w112:refnum<vi>)
        n70 = control-ref of="Col array"() -> (w116:refnum<vi>)
        n71 = control-ref of="Select Layout"() -> (w113:refnum<vi>)
        n72 = Unbundle By Name(w120) -> ("Ctrl"=w119:bool)
        n73 = call "ModeFromDevices.vi"("Devices queue"=w110) -> ("Mode Col"=w111:i32)  [unwired: 9 in, 1 out]
        n74 = control-ref of="Clipboard"() -> (w117:refnum<vi>)
        n75 = case shown="118" w122 {
          tunnel: [w125 w128 eventvkey."Enter" ("VKey") w138 w170] -> w123
          tunnel: w121 -> [w125 w127 _ w137 w169]
          tunnel: w119 -> [_ _ _ w139 w171]
          tunnel: w118 -> [_ _ _ w136 w168]
          tunnel: w114 -> [w124 w126 w131 w135 w167]
          tunnel: w117 -> [_ _ _ w134 w166]
          tunnel: w116 -> [_ _ _ _ w165]
          tunnel: [w124 w126 w131 w133 w164] -> w115
          tunnel: w113 -> [_ _ _ _ w163]
          tunnel: w111 -> [_ _ _ _ w162]
          tunnel: w112 -> [_ _ _ _ w161]
          frame Default {
          }
          frame 0 {
            # "Choose how to handle \"navigation\" keys.\nchar0: arrow keys, enter, return, Shift, Caps, Insert, Ctrl, F-keys"
            n76 = case shown="\"Return\"" w127 {
              selector: w127 -> [w129 _]
              tunnel: [w129 eventvkey."Enter" ("VKey")] -> w128
              frame Default {
              }
              frame "Return" {
                # "Enter (char 0) = num pad key, accept value (remove key focus)\nReturn (char 0) = keyboard enter, edit next."
              }
            }
          }
          frame 9 {
            # "Tab, shift+Tab (char 9) = move edit to right, left.\nSet to Enter to discard \"edit movement\":"
          }
          frame 99 {
            # "c = ASCII char 99: Copy selected cells to clipboard if selection exists."
            n77 = case shown="True" w139 {
              tunnel: [w141 w144] -> w138
              tunnel: w137 -> [w141 w143]
              tunnel: w136 -> [_ w153]
              tunnel: w135 -> [w140 w152]
              tunnel: w134 -> [_ w145]
              tunnel: [w140 w142] -> w133
              frame False {
                # "CTRL not pressed (pass along c-press!)"
              }
              frame True {
                # "non-zero selection?"
                # "user pressed CTRL-C"
                n78 = property class="Tbl (strict)"(reference=w153, error in=w152) -> (reference out=w146:refnum<vi>, error out=w147:errorcluster, "Selection Size"=w150:T5)
                n79 = Greater Than 0?(x=w150) -> (x > 0?=w149:cluster{"Row":bool, "Column":bool})
                n80 = Cluster To Array(cluster=w149) -> (array=w151:bool[])
                n81 = And Array Elements(Boolean array=w151) -> (logical AND=w148:bool)
                n82 = case shown="False" w148 {
                  tunnel: w147 -> [w154 w160]
                  tunnel: w146 -> [_ w159]
                  tunnel: w145 -> [_ w158]
                  tunnel: [w155 w157] -> w144
                  tunnel: w143 -> [w155 w157]
                  tunnel: [w154 w156] -> w142
                  frame False {
                    # "no selection present"
                  }
                  frame True {
                    # "copy selection"
                    n83 = call "CopySelectedCells.vi"("Clipboard"=w158, "error in (no error)"=w160, "Table CtlRef In"=w159) -> ("error out"=w156:errorcluster)  [unwired: 7 in, 1 out]
                  }
                }
              }
            }
          }
          frame 118 {
            # "v = ASCII char 118: Copy selected cells to clipboard if selection exists."
            n84 = case shown="True" w171 {
              tunnel: [w173 w181] -> w170
              tunnel: w169 -> [w173 w180]
              tunnel: w168 -> [_ w190]
              tunnel: w167 -> [w172 w189]
              tunnel: w166 -> [_ w182]
              tunnel: w165 -> [_ w179]
              tunnel: [w172 w177] -> w164
              tunnel: w163 -> [_ w176]
              tunnel: w162 -> [_ w175]
              tunnel: w161 -> [_ w174]
              frame False {
                # "CTRL not pressed (pass along c-press!)"
              }
              frame True {
                # "non-zero selection?"
                # "user pressed CTRL-V"
                n85 = property class="Tbl (strict)"(reference=w190, error in=w189) -> (reference out=w183:refnum<vi>, error out=w184:errorcluster, "Selection Size"=w187:T5, "Selection Start"=w178:T5)
                n86 = Greater Than 0?(x=w187) -> (x > 0?=w186:cluster{"Row":bool, "Column":bool})
                n87 = Cluster To Array(cluster=w186) -> (array=w188:bool[])
                n88 = And Array Elements(Boolean array=w188) -> (logical AND=w185:bool)
                n89 = case shown="True" w185 {
                  tunnel: w184 -> [w191 w202]
                  tunnel: w183 -> [_ w201]
                  tunnel: w182 -> [_ w200]
                  tunnel: [w192 w199] -> w181
                  tunnel: w180 -> [w192 w199]
                  tunnel: w179 -> [_ w198]
                  tunnel: w178 -> [_ w197]
                  tunnel: [w191 w196] -> w177
                  tunnel: w176 -> [_ w195]
                  tunnel: w175 -> [_ w194]
                  tunnel: w174 -> [_ w193]
                  frame False {
                    # "no selection present"
                  }
                  frame True {
                    # "paste selection"
                    n90 = call "PasteSelectedCells.vi"("ModeCol Index"=w194, "Layout Ref"=w195, "Clipboard"=w200, "Table History ref"=w193, "error in (no error)"=w202, "Table CtlRef In"=w201, "Cell Start"=w197, "Col Array Ref in"=w198) -> ("error out"=w196:errorcluster)  [unwired: 1 in, 2 out]
                  }
                }
              }
            }
          }
        }
        n91 = event-data("VKey"=w123) -> ()  [unwired: 6 in, 1 out]
      }
      event "SetList Table": Mouse Down? {
        # "Note: need to check comments in shortcut menu events and update \"mouse down?\" references to new event."
        # "Filter Mouse Down click so that (1) columns can choose to change button (like mode column) and (2) so that some clicks can (sparingly!) be discarded.\nEach column will provide a MouseDown method.\n\nSortClicks (which ultimately called LeftClick) will be moved to Mouse Up event. (is this possible? if shortcut menu is activated, Mouse Up is skipped!)"
        # "No need for DeferPanUpdts here... In fact it screws up click-and-drag!"
        n92 = event-data() -> ("CtlRef"=w221:refnum<vi>, "Coords"=w220:T13, "Button"=w219:u16, "Mods"=w218:cluster{"Double Click":bool, "Menu Key":bool}, "PlatMods"=w217:T16)  [unwired: 1 in]
        "Button\n(Mouse Down?)" <- w219
        n93 = Bundle By Name(cluster=T12 {"CtlRef"=refnum, "Coords"={"Horizontal"=0, "Vertical"=0}, "Button"=0, "Mods"={"Double Click"=FALSE, "Menu Key"=FALSE}, "PlatMods"={"Shift"=FALSE, "Ctrl"=FALSE, "Alt"=FALSE, "Cmd"=FALSE, "Opt"=FALSE}} ("ClickEvent"), "CtlRef"=w221, "Coords"=w220, "Button"=w219, "Mods"=w218, "PlatMods"=w217) -> (w208:T12)
        n94 = local read "Col array"() -> (w213:refnum<class "Column.lvclass">[])
        n95 = control-ref of="Table History"() -> (w209:refnum<vi>)
        n96 = call "SortClicks.vi"("Table History ref"=w209, "error in (no error)"=w216, "ClickEvent in"=w208, "Col array in"=w213) -> ("error out"=w215:errorcluster, "Row Type"=w211:T6, "Click out"=w207:T17, "Col array out"=w212:refnum<class "Column.lvclass">[], "Update HWI?"=w210:bool, "withinData?"=→"withinData?":bool)  [unwired: 2 in]
        n97 = disable-structure shown="Disabled" {
          disable-tunnel: w212 -> [w223 _]
          frame Disabled {
            n98 = local write "Col array"(w223) -> ()
          }
          frame Enabled {
          }
        }
        n99 = case shown="True" w210 {
          frame False {
          }
          frame True {
            n100 = property on="UpdateHWI Button" class="Bool (strict)"("DisabledEnum"=T10."Enabled" ("Disabled")) -> ()  [unwired: 2 in, 2 out]
          }
        }
        n101 = local write "row type"(w211) -> ()
        n102 = Unbundle By Name(w207) -> ("Button"=w205:u16, "Mods"=w204:cluster{"Double Click":bool, "Menu Key":bool}, "PlatMods"=w203:T16, "Discard?"=w206:bool)
        n103 = event-data("Button"=w205, "Mods"=w204, "PlatMods"=w203, "Discard?"=w206) -> ()  [unwired: 1 in, 1 out]
      }
      event "SetList Table": Mouse Up {
        # "Mouse Up is now where the action happens. If up occurs over the same cell as down, it is a \"click\" and left click is called after sorting buttions.\nHowever if up occurs over a different cell than down, we do nothing and let LabVIEW give click-and-drag selection for FREE! Of course, we still\nneed to coerce selection to be within data bounds."
        n104 = event-data() -> ("CtlRef"=w232:refnum<vi>)  [unwired: 1 in, 4 out]
        n105 = property class="Tbl (strict)"(reference=w232, error in=w231) -> (reference out=w227:refnum<vi>, error out=w226:errorcluster, "Selection Size"=w225:T5)
        n106 = Greater Than 0?(x=w225) -> (x > 0?=w230:cluster{"Row":bool, "Column":bool})
        n107 = Cluster To Array(cluster=w230) -> (array=w229:bool[])
        n108 = And Array Elements(Boolean array=w229) -> (logical AND=w228:bool)
        n109 = case shown="True" w228 {
          tunnel: w227 -> [_ w251]
          tunnel: w226 -> [_ w250]
          tunnel: w225 -> [_ w242]
          frame False {
            # "no selection, do nothing."
          }
          frame True {
            # "Force User selection is within data bounds"
            n110 = property class="Tbl (strict)"(reference=w251, error in=w250) -> (reference out=w246:refnum<vi>, error out=w245:errorcluster, "Value"=w248:string[][], "Selection Start"=w249:T5)
            n111 = Add(x=w249, y=w242) -> (x+y=w247:T5)
            n112 = Cluster To Array(cluster=w247) -> (array=w233:i32[])
            n113 = Array Size(array=w248) -> (size(s)=w234:i32[])
            n114 = Subtract(x=w234, y=w233) -> (x-y=w243:i32[])
            n115 = for {
              tunnel: w243 -> [w252] mode=indexing
              tunnel: [w253] -> w241 mode=indexing
              # "coerce"
              n116 = Greater Or Equal To 0?(x=w252) -> (x >= 0?=w254:bool)
              n117 = case shown="False" w254 {
                tunnel: [w255 0] -> w253
                tunnel: w252 -> [w255 _]
                frame False {
                }
                frame True {
                }
              }
            }
            n118 = Unbundle By Name(w242) -> ("Row"=w235:i32, "Column"=w236:i32)
            n119 = Index Array(array=w241) -> (element #1=w238:i32, element #2=w237:i32)  [unwired: 2 in]
            n120 = Add(x=w238, y=w235) -> (x+y=w240:i32)
            n121 = Add(x=w237, y=w236) -> (x+y=w239:i32)
            n122 = Bundle By Name(cluster=w242, "Row"=w240, "Column"=w239) -> (w244:T5)
            n123 = property class="Tbl (strict)"(reference=w246, error in=w245, "Selection Size"=w244) -> ()  [unwired: 2 out]
          }
        }
      }
      event "SetList Table": Shortcut Menu Activation? {
        # "Again, only ModeCol/MenuBuild method needs to write back.\nThis is paied with SortClicks:ModeCol/LeftClick write."
        # "No need for DeferPanUpdts here..."
        # "click within selection?"
        # "#ToDo: Does LMenu have to update col array? (i.e. use private data)"
        # "put active column on shift register?"
        # "row type set after determining click is in a \nvalid column. (Mouse down? event)"
        # "Removed all right-clicks that aren't in a data column\nin Mouse Down? event..."
        n124 = event-data() -> ("CtlRef"=w279:refnum<vi>, "Coords"=w278:T13, "MenuRef"=w266:refnum<k9>)  [unwired: 1 in]
        n125 = invoke class="Tbl (strict)" method="Point To Row Column"(reference=w279, error in=w280, "Point"=w278) -> (reference out=w270:refnum<vi>, error out=w268:errorcluster, "CellPosition"=w264:T5)  [unwired: 3 in, 3 out]
        n126 = Unbundle By Name(w264) -> ("Column"=w276:i32)
        n127 = local read "Col array"() -> (w258:refnum<class "Column.lvclass">[])
        n128 = property class="Tbl (strict)"(reference=w270, error in=w268) -> (reference out=w269:refnum<vi>, error out=w267:errorcluster, "Selection Size"=w265:T5, "Selection Start"=w263:T5)
        n129 = Index Array(array=w258, index=w276) -> (element=w277:refnum<class "Column.lvclass">)
        n130 = Add(x=w265, y=w263) -> (x+y=w273:T5)
        n131 = local read "Button\n(Mouse Down?)"() -> (w257:u16)
        n132 = control-ref of="Clipboard"() -> (w259:refnum<vi>)
        n133 = Greater?(x=w273, y=w264) -> (0:w272:cluster{"Row":bool, "Column":bool})
        n134 = Less Or Equal?(x=w263, y=w264) -> (x <= y?=w271:cluster{"Row":bool, "Column":bool})
        n135 = And(x=w272, y=w271) -> (x .and. y?=w262:cluster{"Row":bool, "Column":bool})
        n136 = Cluster To Array(cluster=w262) -> (array=w261:bool[])
        n137 = And Array Elements(Boolean array=w261) -> (logical AND=w260:bool)
        "withinSelection?" <- w260
        n138 = call-dynamic "MenuBuild.vi"("Button\n(Mouse Down?)"=w257, "Clipboard"=w259, "withinSelection?"=w260, "row type"="row type", "error in (no error)"=w267, "Table CtlRef In"=w269, "MenuRef In"=w266, "Column in"=w277) -> ("error out"=w281:errorcluster, "Column out"=w275:refnum<class "Column.lvclass">)  [unwired: 2 out]
        n139 = disable-structure shown="Disabled" {
          disable-tunnel: w276 -> [w285 _]
          disable-tunnel: w275 -> [w284 _]
          disable-tunnel: w258 -> [w282 _]
          frame Disabled {
            # "update col array"
            n140 = Replace Array Subset(array=w282, new element=w284, index=w285) -> (w283:refnum<class "Column.lvclass">[])
            n141 = local write "Col array"(w283) -> ()
          }
          frame Enabled {
          }
        }
        n142 = event-data() -> ()  [unwired: 2 in, 1 out]
      }
      event "SetList Table": Shortcut Menu Selection (User) {
        # "Don't check error or panel it\nmay prevent panel being updated!"
        # "all columns needed for certain actions \n(e.g. maser mode change, show hidden columns)"
        n143 = event-data() -> ("CtlRef"=w291:refnum<vi>, "Coords"=w309:T13, "ItemTag"=w308:string)  [unwired: 1 in, 2 out]
        n144 = invoke class="Tbl (strict)" method="Point To Row Column"(reference=w291, error in=w310, "Point"=w309) -> (reference out=w290:refnum<vi>, error out=w295:errorcluster, "CellPosition"=w307:T5)  [unwired: 3 in, 3 out]
        n145 = local read "Defer Updates?"() -> (w292:bool)
        n146 = call "DefPnlAndCursor.vi"("AllowDefPan? (T)"=w292, "error in (no error)"=w295, "DeferPanUpdts?"=TRUE ("DeferPanUPdts?"), "Tbl Ctrl Refnum"=w290) -> ("error out"=w301:errorcluster)  [unwired: 7 in]
        n147 = control-ref of="VariableManager"() -> (w289:refnum<vi>)
        n148 = local read "Devices queue"() -> (w287:refnum<queue>)
        n149 = local read "Col array"() -> (w306:refnum<class "Column.lvclass">[])
        n150 = call "ModeFromDevices.vi"("Devices queue"=w287) -> ("Mode Col"=w288:i32)  [unwired: 9 in, 1 out]
        n151 = Unbundle By Name(w307) -> ("Column"=w303:i32)
        n152 = control-ref of="Col array"() -> (w297:refnum<vi>)
        n153 = control-ref of="Select Layout"() -> (w296:refnum<vi>)
        n154 = Index Array(array=w306, index=w303) -> (element=w305:refnum<class "Column.lvclass">)
        n155 = control-ref of="Table History"() -> (w300:refnum<vi>)
        n156 = control-ref of="Clipboard"() -> (w302:refnum<vi>)
        n157 = call-dynamic "MenuDo.vi"("Column in"=w305, "Col Array Ref in"=w297, "Layout Ring Refnum"=w296, "Clipboard"=w302, "ItemTag"=w308, "VariableManagerRef"=w289, "Table CtlRef In"=w290, "error in (no error)"=w301, "Cell Position"=w307, "ModeCol Index"=w288, "Table History ref"=w300) -> ("Column out"=w304:refnum<class "Column.lvclass">, "Update HWI?"=w286:bool, "error out"=w299:errorcluster)  [unwired: 2 out]
        n158 = disable-structure shown="Disabled" {
          disable-tunnel: w304 -> [w312 _]
          disable-tunnel: w303 -> [w311 _]
          frame Disabled {
            # "update col array"
            n159 = local read "Col array"() -> (w313:refnum<class "Column.lvclass">[])
            n160 = Replace Array Subset(array=w313, new element=w312, index=w311) -> (w314:refnum<class "Column.lvclass">[])
            n161 = local write "Col array"(w314) -> ()
          }
          frame Enabled {
          }
        }
        n162 = case shown="True" w286 {
          frame False {
          }
          frame True {
            n163 = property on="UpdateHWI Button" class="Bool (strict)"("DisabledEnum"=T10."Enabled" ("Disabled")) -> ()  [unwired: 2 in, 2 out]
          }
        }
        n164 = call "DefPnlAndCursor.vi"("AllowDefPan? (T)"=w292, "error in (no error)"=w299, "DeferPanUpdts?"=FALSE ("DeferPanUPdts?"), "Tbl Ctrl Refnum"=w290) -> ("error out"=w298:errorcluster)  [unwired: 7 in]
      }
      event "SetList Table": Mouse Enter {
        # "Change to hand inside table"
        n165 = event-data() -> ()  [unwired: 1 in, 1 out]
        n166 = call-poly <vilib>:"Set Cursor.vi"("error in (no error)"=w317, "icon"=6) -> ("error out"=w316:errorcluster)  [unwired: 8 in, 1 out]
      }
      event "SetList Table": Mouse Leave {
        # "Change back to default pointer outside table control"
        n167 = event-data() -> ()  [unwired: 1 in, 1 out]
        n168 = call-poly <vilib>:"Set Cursor.vi"("error in (no error)"=w320, "icon"=0) -> ("error out"=w319:errorcluster)  [unwired: 8 in, 1 out]
      }
      event "User defined functions": Value Change {
        n169 = event-data() -> ("OldVal"=w323:string, "NewVal"=w322:string)  [unwired: 1 in, 1 out]
        n170 = call "Caching_Expression_Evaluator_v4.vi"("method"=t_Caching_Expression_Evaluator_Methods_v4."execute", "expression/scriptlet"=w322, "error in (no error)"=w325) -> ("error out"=w326:errorcluster)  [unwired: 11 in, 1 out]
        n171 = case shown="No Error" w326 {
          selector: w326 -> [w329 w331]
          tunnel: [w329 errorcluster {"status"=FALSE, "code"=0, "source"=""} ("error out")] -> w324
          tunnel: w323 -> [_ w332]
          tunnel: w322 -> [w328 _]
          frame No Error {
            n172 = global write "NextMaster_v4.vi" "User Procedures"(w328) -> ()
          }
          frame Error {
            # "on parsing error: reset functions to last, Clear error (and present warning dialog)"
            n173 = local write "User defined functions"(w332) -> ()
            n174 = disable-structure shown="Enabled" {
              disable-tunnel: w331 -> [w336 _]
              frame Enabled {
                w338 = T18 1 items=["no dialog", "OK message", "continue or stop message", "OK message + warnings", "continue/stop + warnings"] ("type of dialog (OK msg:1)")
                n175 = Unbundle By Name(w336) -> ("source"=w334:string)
                n176 = Concatenate Strings("\n*User Functions* error: \n" ("string"), w334) -> (w335:string)
                n177 = Bundle By Name(cluster=w336, "source"=w335) -> (w337:errorcluster)
                n178 = call <vilib>:"Simple Error Handler.vi"("type of dialog (OK msg:1)"=w338, "error in (no error)"=w337) -> ()  [unwired: 3 in, 5 out]
              }
              frame Disabled {
              }
            }
          }
        }
      }
      event "Select Layout": Value Change {
        n179 = event-data() -> ("NewVal"=w349:i32)  [unwired: 1 in, 2 out]
        n180 = local read "Defer Updates?"() -> (w339:bool)
        n181 = call "DefPnlAndCursor.vi"("AllowDefPan? (T)"=w339, "error in (no error)"=w344, "DeferPanUpdts?"=TRUE ("DeferPanUPdts?"), "Tbl Ctrl Refnum"=w340) -> ("error out"=w345:errorcluster)  [unwired: 7 in]
        n182 = local read "Col array"() -> (w347:refnum<class "Column.lvclass">[])
        n183 = control-ref of="SetList Table"() -> (w348:refnum<vi>)
        n184 = call "ApplySelectedLayout.vi"("error in (no error)"=w345, "Layout index"=w349, "Col array"=w347, "Tbl Refnum"=w348) -> ("error out"=w342:errorcluster)  [unwired: 7 in]
        n185 = call "DefPnlAndCursor.vi"("AllowDefPan? (T)"=w339, "error in (no error)"=w342, "DeferPanUpdts?"=FALSE ("DeferPanUPdts?"), "Tbl Ctrl Refnum"=w340) -> ("error out"=w341:errorcluster)  [unwired: 7 in]
      }
      event "ConfigLayoutsButton": Value Change {
        # "Make sure col array is updated \nwith \"filmstrip\" sequence!"
        # "Want preview of layouts as we make them\n-->VI gets panel reference from table control to defer updates as required."
        n186 = event-data() -> ()  [unwired: 1 in, 3 out]
        n187 = disable-structure shown="Enabled" {
          frame Enabled {
            # "reset button"
            n188 = local write "ConfigLayoutsButton"(FALSE) -> ()
          }
          frame Disabled {
          }
        }
        n189 = flat-sequence {
          tunnel: w352 -> [w358]
          tunnel: [w353] -> w351
          tunnel: [w362] -> w350
          tunnel: w351 -> [w363]
          frame #0 {
            n190 = local read "Defer Updates?"() -> (w355:bool)
            n191 = control-ref of="Select Layout"() -> (w356:refnum<vi>)
            n192 = control-ref of="Col array"() -> (w354:refnum<vi>)
            n193 = control-ref of="SetList Table"() -> (w357:refnum<vi>)
            n194 = call "ConfigLayouts.vi"("Defer Updates? (True)"=w355, "Tbl Refnum"=w357, "error in (no error)"=w358, "Col Array Refnum"=w354, "Layout Ring Refnum"=w356) -> ("error out"=w353:errorcluster)  [unwired: 6 in]
          }
          frame #1 {
            # "Need to push appearance changes\nto the columns! (or change layout\nto act on devices...)"
            n195 = local read "Devices queue"() -> (w359:refnum<queue>)
            n196 = local read "Col array"() -> (w361:refnum<class "Column.lvclass">[])
            n197 = local read "DevNums"() -> (w360:i32[])
            n198 = call "SetList Columns to Devices.vi"("error in (no error)"=w363, "Col array in"=w361, "DevNums In"=w360, "Devices queue"=w359) -> ("error out"=w362:errorcluster)  [unwired: 6 in, 1 out]
          }
        }
      }
      event "FitCol2Text Button": Value Change {
        # "Resizes all displayed columns"
        n199 = event-data() -> ()  [unwired: 1 in, 3 out]
        n200 = local read "Defer Updates?"() -> (w366:bool)
        n201 = local read "SetList Table"() -> (w378:string[][])
        n202 = local read "Col array"() -> (w374:refnum<class "Column.lvclass">[])
        n203 = local read "Select Layout"() -> (w373:i32)
        n204 = property on="SetList Table" class="Tbl (strict)"() -> ("Column Headers[]"=w375:string[])  [unwired: 2 in, 2 out]
        n205 = call "DefPnlAndCursor.vi"("AllowDefPan? (T)"=w366, "error in (no error)"=w368, "DeferPanUpdts?"=TRUE ("DeferPanUPdts?"), "Tbl Ctrl Refnum"=w367) -> ("error out"=w369:errorcluster)  [unwired: 7 in]
        n206 = Transpose 2D Array(2D array=w378) -> (transposed array=w376:string[][])
        n207 = for {
          tunnel: w376 -> [w389] mode=indexing
          shift-right: [w386] -> w370
          shift-left: w369 -> [w387]
          tunnel: w375 -> [w385] mode=indexing
          tunnel: w374 -> [w384] mode=indexing
          tunnel: w373 -> [w379]
          i -> [w388]
          n208 = call "GetLayoutInfo.vi"("Column in"=w384) -> ("Layout cluster"=w381:T19)  [unwired: 8 in, 2 out]
          n209 = Unbundle By Name(w381) -> ("Width"=w382:u32, "[disp?]"=w380:bool[])
          n210 = case shown="Default" w379 {
            selector: w379 -> [_ w391]
            tunnel: [TRUE ("Displayed?") w393] -> w383
            tunnel: w380 -> [_ w392]
            frame ..-1 {
            }
            frame Default {
              n211 = Index Array(array=w392, index=w391) -> (element=w393:bool)
            }
          }
          n212 = case shown="True" w383 {
            tunnel: w389 -> [_ w410]
            tunnel: w388 -> [_ w408]
            tunnel: w387 -> [w394 w401]
            tunnel: [w394 w406] -> w386
            tunnel: w385 -> [_ w402]
            tunnel: w382 -> [_ w395]
            frame False {
            }
            frame True {
              # "Don't show hidden\ncolumns (alreay have\nwidth=0)\nNote: will not respect \n\"on-the-fly\" hiding"
              n213 = for {
                shift-right: [w414] -> w405
                shift-left: 0 -> [w416]
                tunnel: w410 -> [w413] mode=indexing
                n214 = call <vilib>:"Get Text Rect.vi"("text"=w413) -> ("rect"=w417:T20)  [unwired: 8 in]
                n215 = Unbundle By Name(w417) -> ("right"=w415:i16)
                n216 = Max & Min(x=w416, y=w415) -> (max(x,y)=w414:i32)  [unwired: 1 out]
              }
              n217 = call <vilib>:"Get Text Rect.vi"("text"=w402) -> ("rect"=w404:T20)  [unwired: 8 in]
              n218 = Unbundle By Name(w404) -> ("right"=w403:i16)
              n219 = Max & Min(x=w405, y=w403) -> (max(x,y)=w398:i32)  [unwired: 1 out]
              n220 = Not Equal To 0?(x=w395) -> (x != 0?=w397:bool)
              n221 = Add(x=w398, y=8) -> (x+y=w400:i32)
              n222 = Bundle("Row"=-2, w408) -> (w407:cluster{"Row":i32, i32})  [unwired: 1 in]
              n223 = Select(t=w400, s=w397, f=0 ("y")) -> (s? t:f=w399:i32)
              n224 = property on="SetList Table" class="Tbl (strict)"(error in=w401, "Active Cell"=w407, "Width"=w399) -> (error out=w406:errorcluster)  [unwired: 1 in, 1 out]
            }
          }
        }
        n225 = local write "FitCol2Text Button"(FALSE ("FitCol2Text Button")) -> ()
        n226 = call "DefPnlAndCursor.vi"("AllowDefPan? (T)"=w366, "error in (no error)"=w370, "DeferPanUpdts?"=FALSE ("DeferPanUPdts?"), "Tbl Ctrl Refnum"=w367) -> ("error out"=w365:errorcluster)  [unwired: 7 in]
      }
      event Value Change {
        # "Add Device is also used in Manage Devices.vi, so it was simpler\nto leave it expecting the [Devices] and dequeue-enqueue around it."
        # "Note: DevNums are used in \"Device Change to SetList.vi\""
        # "Converted to subVI so Manage can use same code for Add!"
        n227 = event-data() -> ("CtlRef"=w445:refnum<vi>)  [unwired: 1 in, 2 out]
        n228 = local read "Defer Updates?"() -> (w427:bool)
        n229 = call "DefPnlAndCursor.vi"("AllowDefPan? (T)"=w427, "error in (no error)"=w428, "DeferPanUpdts?"=TRUE ("DeferPanUPdts?"), "Tbl Ctrl Refnum"=w426) -> ("error out"=w429:errorcluster)  [unwired: 7 in]
        n230 = control-ref of="SetList Table"() -> (w438:refnum<vi>)
        n231 = property class="Tbl (strict)"(reference=w438, error in=w429) -> (reference out=w433:refnum<vi>, error out=w437:errorcluster, "Value"=w436:string[][])
        n232 = local read "Devices queue"() -> (w435:refnum<queue>)
        n233 = local read "DevNums"() -> (w434:i32[])
        n234 = local read "Col array"() -> (w444:refnum<class "Column.lvclass">[])
        n235 = control-ref of="Table History"() -> (w439:refnum<vi>)
        n236 = call "SetList SWI to Devices.vi"("error in (no error)"=w437, "SWI table"=w436, "DevNums In"=w434, "Devices queue"=w435) -> ("error out"=w423:errorcluster, "Devices queue out"=w425:refnum<queue>)  [unwired: 5 in, 1 out]
        n237 = Dequeue Element(queue=w425, error in (no error)=w423) -> (queue out=w421:refnum<queue>, element=w422:refnum<class "Device.lvclass">[], error out=w424:errorcluster)  [unwired: 1 in, 1 out]
        n238 = control-ref of="Select Layout"() -> (w441:refnum<vi>)
        n239 = call "AddDevice.vi"("Device List in"=w422, "Table Ref In"=w433, "Table History ref"=w439, "Layout Ref"=w441, "DevNums In"=w434, "Col array in"=w444, "error in (no error)"=w424, "Add Device"=w445) -> ("Device List out"=w418:refnum<class "Device.lvclass">[], "DevNums Out"=w442:i32[], "Col array out"=w443:refnum<class "Column.lvclass">[], "Changes Made?"=w440:bool, "error out"=w420:errorcluster)  [unwired: 3 in]
        n240 = local write "DevNums"(w442) -> ()
        n241 = Enqueue Element(queue=w421, element=w418, error in (no error)=w420) -> (error out=w419:errorcluster)  [unwired: 1 in, 2 out]
        n242 = local write "Col array"(w443) -> ()
        n243 = call "DefPnlAndCursor.vi"("AllowDefPan? (T)"=w427, "error in (no error)"=w419, "DeferPanUpdts?"=FALSE ("DeferPanUPdts?"), "Tbl Ctrl Refnum"=w426) -> ("error out"=w431:errorcluster)  [unwired: 7 in]
        n244 = case shown="True" w440 {
          frame False {
          }
          frame True {
            n245 = property on="UpdateHWI Button" class="Bool (strict)"("DisabledEnum"=T10."Enabled" ("Disabled")) -> ()  [unwired: 2 in, 2 out]
          }
        }
      }
      event "ManageDevicesButton": Value Change {
        # "push SWI to devices (so they can operate\non it easily if column #s change)"
        n246 = event-data() -> ()  [unwired: 1 in, 3 out]
        n247 = control-ref of="SetList Table"() -> (w455:refnum<vi>)
        n248 = property class="Tbl (strict)"(reference=w455) -> (reference out=w454:refnum<vi>, error out=w452:errorcluster, "Value"=w451:string[][])  [unwired: 1 in]
        n249 = local read "Devices queue"() -> (w450:refnum<queue>)
        n250 = local read "DevNums"() -> (w453:i32[])
        n251 = call "SetList SWI to Devices.vi"("error in (no error)"=w452, "SWI table"=w451, "DevNums In"=w453, "Devices queue"=w450) -> ("Devices queue out"=w447:refnum<queue>)  [unwired: 5 in, 2 out]
        n252 = local read "DevNums"() -> (w460:i32[])
        n253 = local read "Col array"() -> (w459:refnum<class "Column.lvclass">[])
        n254 = control-ref of="Table History"() -> (w448:refnum<vi>)
        n255 = local write "ManageDevicesButton"(FALSE) -> ()
        n256 = control-ref of="Select Layout"() -> (w456:refnum<vi>)
        n257 = call "Manage Devices.vi"("Devices queue"=w447, "Table Ref In"=w454, "DevNums In"=w460, "Col array in"=w459, "Table History ref"=w448, "Layout ref"=w456) -> ("Changes Made?"=w449:bool, "DevNums Out"=w457:i32[], "Col array out"=w458:refnum<class "Column.lvclass">[])  [unwired: 1 in, 1 out]
        n258 = local write "DevNums"(w457) -> ()
        n259 = local write "Col array"(w458) -> ()
        n260 = case shown="True" w449 {
          frame False {
          }
          frame True {
            n261 = property on="UpdateHWI Button" class="Bool (strict)"("DisabledEnum"=T10."Enabled" ("Disabled")) -> ()  [unwired: 2 in, 2 out]
          }
        }
      }
      event "quit": Value Change {
        # "store devices state on Quit.\nThis should be the ONLY local variable call!!!"
        # "Save SWI to device array. If VI is restarted, the table will be re-initialized\nfrom device array, erasing any bug-causing user edits to table control\nthe user made while VI was stopped."
        # "Stop VMUI when stopping SetList (otherwise Actor stays in memory until LabView closed.)"
        n262 = event-data() -> ("NewVal"=w477:bool)  [unwired: 1 in, 1 out]
        n263 = control-ref of="VariableManager"() -> (w469:refnum<vi>)
        n264 = control-ref of="SetList Table"() -> (w476:refnum<vi>)
        n265 = property class="Tbl (strict)"(reference=w476, error in=w471) -> (error out=w474:errorcluster, "Value"=w473:string[][])  [unwired: 1 out]
        n266 = local read "Devices queue"() -> (w472:refnum<queue>)
        n267 = local read "DevNums"() -> (w475:i32[])
        n268 = call "VMUIStop.vi"("VariableManagerRef in"=w469) -> ()  [unwired: 9 in, 2 out]
        n269 = call "SetList SWI to Devices.vi"("error in (no error)"=w474, "SWI table"=w473, "DevNums In"=w475, "Devices queue"=w472) -> ("error out"=w466:errorcluster, "Devices queue out"=w467:refnum<queue>)  [unwired: 5 in, 1 out]
        n270 = Dequeue Element(queue=w467, error in (no error)=w466) -> (queue out=w465:refnum<queue>, element=w463:refnum<class "Device.lvclass">[], error out=w464:errorcluster)  [unwired: 1 in, 1 out]
        n271 = local write "Devices"(w463) -> ()
        n272 = Release Queue(queue=w465, error in (no error)=w464) -> (error out=w468:errorcluster)  [unwired: 1 in, 2 out]
        n273 = local write "quit"(FALSE ("quit")) -> ()
      }
      event "Undo": Value Change {
        n274 = event-data() -> ()  [unwired: 1 in, 3 out]
        n275 = local read "Defer Updates?"() -> (w481:bool)
        n276 = disable-structure shown="Enabled" {
          disable-tunnel: [w496 w498] -> w483
          disable-tunnel: w482 -> [w495 w498]
          disable-tunnel: w481 -> [w494 _]
          disable-tunnel: w480 -> [w493 _]
          frame Enabled {
            n277 = call "DefPnlAndCursor.vi"("AllowDefPan? (T)"=w494, "error in (no error)"=w495, "DeferPanUpdts?"=TRUE ("DeferPanUPdts?"), "Tbl Ctrl Refnum"=w493) -> ("error out"=w496:errorcluster)  [unwired: 7 in]
          }
          frame Disabled {
          }
        }
        n278 = local read "Devices queue"() -> (w478:refnum<queue>)
        n279 = local read "Col array"() -> (w489:refnum<class "Column.lvclass">[])
        n280 = control-ref of="Table History"() -> (w491:refnum<vi>)
        n281 = control-ref of="SetList Table"() -> (w492:refnum<vi>)
        n282 = call "ModeFromDevices.vi"("Devices queue"=w478) -> ("Mode Col"=w479:i32)  [unwired: 9 in, 1 out]
        n283 = local write "Undo"(FALSE ("Undo")) -> ()
        n284 = control-ref of="Select Layout"() -> (w488:refnum<vi>)
        n285 = call "Un(Re)doTblChng.vi"("Undo/Redo"=enum16{"Undo", "Redo"}."Undo", "ModeCol Index"=w479, "Layout Ref"=w488, "error in (no error)"=w483, "Table CtlRef In"=w492, "Col Array in"=w489, "Table History ref"=w491) -> ("error out"=w485:errorcluster)  [unwired: 4 in]
        n286 = disable-structure shown="Enabled" {
          disable-tunnel: w485 -> [w502 w504]
          disable-tunnel: [w501 w504] -> w484
          disable-tunnel: w481 -> [w500 _]
          disable-tunnel: w480 -> [w499 _]
          frame Enabled {
            n287 = call "DefPnlAndCursor.vi"("AllowDefPan? (T)"=w500, "error in (no error)"=w502, "DeferPanUpdts?"=FALSE ("DeferPanUPdts?"), "Tbl Ctrl Refnum"=w499) -> ("error out"=w501:errorcluster)  [unwired: 7 in]
          }
          frame Disabled {
          }
        }
        n288 = property on="UpdateHWI Button" class="Bool (strict)"("DisabledEnum"=T10."Enabled" ("Disabled")) -> ()  [unwired: 2 in, 2 out]
      }
      event "Redo": Value Change {
        n289 = event-data() -> ()  [unwired: 1 in, 3 out]
        n290 = local read "Defer Updates?"() -> (w508:bool)
        n291 = disable-structure shown="Enabled" {
          disable-tunnel: w512 -> [w523 w525]
          disable-tunnel: [w522 w525] -> w511
          disable-tunnel: w508 -> [w521 _]
          disable-tunnel: w507 -> [w520 _]
          frame Enabled {
            n292 = call "DefPnlAndCursor.vi"("AllowDefPan? (T)"=w521, "error in (no error)"=w523, "DeferPanUpdts?"=TRUE ("DeferPanUPdts?"), "Tbl Ctrl Refnum"=w520) -> ("error out"=w522:errorcluster)  [unwired: 7 in]
          }
          frame Disabled {
          }
        }
        n293 = local read "Devices queue"() -> (w506:refnum<queue>)
        n294 = local read "Col array"() -> (w516:refnum<class "Column.lvclass">[])
        n295 = control-ref of="Table History"() -> (w518:refnum<vi>)
        n296 = control-ref of="SetList Table"() -> (w519:refnum<vi>)
        n297 = local write "Redo"(FALSE) -> ()
        n298 = call "ModeFromDevices.vi"("Devices queue"=w506) -> ("Mode Col"=w505:i32)  [unwired: 9 in, 1 out]
        n299 = control-ref of="Select Layout"() -> (w514:refnum<vi>)
        n300 = call "Un(Re)doTblChng.vi"("Undo/Redo"=enum16{"Undo", "Redo"}."Redo", "ModeCol Index"=w505, "Layout Ref"=w514, "error in (no error)"=w511, "Table CtlRef In"=w519, "Col Array in"=w516, "Table History ref"=w518) -> ("error out"=w509:errorcluster)  [unwired: 4 in]
        n301 = disable-structure shown="Enabled" {
          disable-tunnel: [w529 w531] -> w510
          disable-tunnel: w509 -> [w528 w531]
          disable-tunnel: w508 -> [w527 _]
          disable-tunnel: w507 -> [w526 _]
          frame Enabled {
            n302 = call "DefPnlAndCursor.vi"("AllowDefPan? (T)"=w527, "error in (no error)"=w528, "DeferPanUpdts?"=FALSE ("DeferPanUPdts?"), "Tbl Ctrl Refnum"=w526) -> ("error out"=w529:errorcluster)  [unwired: 7 in]
          }
          frame Disabled {
          }
        }
        n303 = property on="UpdateHWI Button" class="Bool (strict)"("DisabledEnum"=T10."Enabled" ("Disabled")) -> ()  [unwired: 2 in, 2 out]
      }
      event "Save to Disk": Value Change {
        n304 = event-data() -> ("NewVal"=w532:bool)  [unwired: 1 in, 2 out]
        n305 = case shown="True" w532 {
          frame False {
          }
          frame True {
            # "Also need to push SWI to devices prior to saving!\nWhat about HWI?"
            n306 = local read "Devices queue"() -> (w539:refnum<queue>)
            n307 = control-ref of="VariableManager"() -> (w535:refnum<vi>)
            n308 = local read "DevNums"() -> (w540:i32[])
            n309 = property on="SetList Table" class="Tbl (strict)"() -> (error out=w537:errorcluster, "Value"=w538:string[][])  [unwired: 2 in, 1 out]
            n310 = local write "Save to Disk"(FALSE ("Load from Disk")) -> ()
            n311 = property on="Select Layout" class="Ring (strict)"() -> ("Value"=w545:i32, "StringsAndValues[]"=w544:T15)  [unwired: 2 in, 2 out]
            n312 = local read "User defined functions"() -> (w543:string)
            n313 = call "SetList SWI to Devices.vi"("error in (no error)"=w537, "SWI table"=w538, "DevNums In"=w540, "Devices queue"=w539) -> ("error out"=w536:errorcluster, "Devices out"=w533:refnum<class "Device.lvclass">[])  [unwired: 5 in, 1 out]
            n314 = call "VMExport.vi"("VariableManagerRef in"=w535) -> ("VariableManagerExportCopy"=w534:refnum<class "VariableManager.lvclass">)  [unwired: 8 in, 2 out]
            n315 = Bundle By Name(cluster=T14 {"Version"="", "Devices"=[], "Select Layout"=0, "Layout:Strings And Values []"=[], "User defined functions"="", "VariableManager"=refnum}, "Version"="testing", "Devices"=w533, "Select Layout"=w545, "Layout:Strings And Values []"=w544, "User defined functions"=w543, "VariableManager"=w534) -> (w541:T14)
            n316 = call "Save_v5.vi"("error in"=w536, "Save Cluster"=w541) -> ("cancelled"=w548:bool, "Procedure Name"=w547:string, "Chosen Path"=w549:path)  [unwired: 6 in, 1 out]
            n317 = case shown="False" w548 {
              tunnel: w549 -> [w552 _]
              tunnel: w547 -> [w551 _]
              frame False {
                # "user saved!"
                n318 = local write "Procedure Name"(w551) -> ()
                n319 = control-ref of="Load Recent"() -> (w553:refnum<vi>)
                n320 = call "Load_HistoryUpdate.vi"("History ref"=w553, "New Path"=w552) -> ()  [unwired: 1 in]
              }
              frame True {
                # "user cancelled"
              }
            }
          }
        }
      }
      event "Load from Disk": Value Change {
        n321 = event-data() -> ("NewVal"=w554:bool)  [unwired: 1 in, 2 out]
        n322 = case shown="True" w554 {
          frame False {
          }
          frame True {
            # "ToDo: This is duplicate code! Change to function which takes control references; reuse on Load... .\nAlso need to initialize table from devices!!!"
            n323 = call "Load_v5.vi"() -> ("error out"=w555:errorcluster, "cancelled"=w560:bool, "Procedure Name"=w558:string, "Chosen Path"=w559:path, "Save Cluster"=w557:T14)  [unwired: 7 in]
            n324 = local write "Load from Disk"(FALSE ("Load from Disk")) -> ()
            n325 = case shown="False" w560 {
              tunnel: w559 -> [w577 _]
              tunnel: w558 -> [w576 _]
              tunnel: w557 -> [w569 _]
              tunnel: w555 -> [w568 _]
              tunnel: [FALSE ("Visible") _] -> w556
              frame False {
                # "user saved!"
                n326 = local write "Procedure Name"(w576) -> ()
                n327 = control-ref of="Load Recent"() -> (w578:refnum<vi>)
                n328 = control-ref of="SetList Table"() -> (w563:refnum<vi>)
                n329 = control-ref of="VariableManager"() -> (w564:refnum<vi>)
                n330 = property on="Loading Text" class="Str"("Visible"=TRUE) -> ()  [unwired: 2 in, 2 out]
                n331 = local read "Defer Updates?"() -> (w572:bool)
                n332 = local read "Devices queue"() -> (w562:refnum<queue>)
                n333 = call "Load_HistoryUpdate.vi"("History ref"=w578, "New Path"=w577) -> ()  [unwired: 1 in]
                n334 = control-ref of="Select Layout"() -> (w570:refnum<vi>)
                n335 = call "LoadedCluster_toSetList_v5.vi"("Devices queue"=w562, "Layout Ref"=w570, "Save Cluster"=w569, "Table Ref in"=w563, "VariableManagerRef"=w564, "error in (no error)"=w568, "Defer Updates? (T)"=w572) -> ("Loaded Version"=w571:string, "DevNums"=w573:i32[], "Col array"=w574:refnum<class "Column.lvclass">[], "User defined functions"=w567:string)  [unwired: 3 in, 2 out]
                n336 = local write "User defined functions"(w567) -> ()
                n337 = global write "NextMaster_v4.vi" "User Procedures"(w567) -> ()
                n338 = local write "Loaded Version"(w571) -> ()
                n339 = property on="UpdateHWI Button" class="Bool (strict)"("DisabledEnum"=T10."Enabled" ("Disabled")) -> ()  [unwired: 2 in, 2 out]
                n340 = local write "DevNums"(w573) -> ()
                n341 = local write "Col array"(w574) -> ()
              }
              frame True {
                # "user cancelled"
              }
            }
            n342 = property on="Loading Text" class="Str"("Visible"=w556) -> ()  [unwired: 2 in, 2 out]
          }
        }
      }
      event "Load Recent": Value Change {
        # "ToDo: This is duplicate code! Change to function which takes control references; reuse on Load... .\nAlso need to initialize table from devices!!!"
        n343 = event-data() -> ("NewVal"=w587:string)  [unwired: 1 in, 2 out]
        n344 = String To Path(string=w587) -> (path=w583:path)
        n345 = call "Load_v5.vi"("Path (open dialog)"=w583) -> ("error out"=w581:errorcluster, "cancelled"=w586:bool, "Procedure Name"=w584:string, "Chosen Path"=w585:path, "Save Cluster"=w580:T14)  [unwired: 6 in]
        n346 = case shown="False" w586 {
          tunnel: w585 -> [w602 _]
          tunnel: w584 -> [w601 _]
          tunnel: w581 -> [w595 _]
          tunnel: w580 -> [w594 _]
          tunnel: [FALSE ("Visible") _] -> w579
          frame False {
            # "user loaded!"
            n347 = control-ref of="SetList Table"() -> (w589:refnum<vi>)
            n348 = control-ref of="VariableManager"() -> (w590:refnum<vi>)
            n349 = local write "Procedure Name"(w601) -> ()
            n350 = control-ref of="Load Recent"() -> (w603:refnum<vi>)
            n351 = local read "Defer Updates?"() -> (w598:bool)
            n352 = local read "Devices queue"() -> (w588:refnum<queue>)
            n353 = control-ref of="Select Layout"() -> (w597:refnum<vi>)
            n354 = call "Load_HistoryUpdate.vi"("History ref"=w603, "New Path"=w602) -> ()  [unwired: 1 in]
            n355 = call "LoadedCluster_toSetList_v5.vi"("Devices queue"=w588, "Layout Ref"=w597, "Save Cluster"=w594, "Table Ref in"=w589, "VariableManagerRef"=w590, "error in (no error)"=w595, "Defer Updates? (T)"=w598) -> ("Loaded Version"=w596:string, "DevNums"=w599:i32[], "Col array"=w600:refnum<class "Column.lvclass">[], "User defined functions"=w593:string)  [unwired: 3 in, 2 out]
            n356 = local write "User defined functions"(w593) -> ()
            n357 = global write "NextMaster_v4.vi" "User Procedures"(w593) -> ()
            n358 = local write "Loaded Version"(w596) -> ()
            n359 = property on="Loading Text" class="Str"("Visible"=TRUE) -> ()  [unwired: 2 in, 2 out]
            n360 = local write "DevNums"(w599) -> ()
            n361 = local write "Col array"(w600) -> ()
          }
          frame True {
            # "user cancelled"
          }
        }
        n362 = property on="Loading Text" class="Str"("Visible"=w579) -> ()  [unwired: 2 in, 2 out]
        n363 = property on="UpdateHWI Button" class="Bool (strict)"("DisabledEnum"=T10."Enabled" ("Disabled")) -> ()  [unwired: 2 in, 2 out]
      }
      event "Load Old": Value Change {
        n364 = event-data() -> ("NewVal"=w605:bool)  [unwired: 1 in, 2 out]
        n365 = case shown="True" w605 {
          tunnel: [_ FALSE ("Load from Disk")] -> w604
          frame False {
          }
          frame True {
            n366 = local read "Old Procedure Path"() -> (w617:path)
            n367 = local read "Version Selection"() -> (w612:T4)
            n368 = local write "Load Old"(FALSE ("Load from Disk")) -> ()
            n369 = property on="Loading Text" class="Str"("Visible"=TRUE ("Load from Disk")) -> ()  [unwired: 2 in, 2 out]
            n370 = control-ref of="Old Procedure History"() -> (w626:refnum<vi>)
            n371 = control-ref of="VariableManager"() -> (w608:refnum<vi>)
            n372 = call "Load_HistoryUpdate.vi"("History ref"=w626, "New Path"=w617) -> ()  [unwired: 1 in]
            n373 = local read "Devices queue"() -> (w606:refnum<queue>)
            n374 = local read "Defer Updates?"() -> (w621:bool)
            n375 = control-ref of="SetList Table"() -> (w607:refnum<vi>)
            n376 = local read "Old HWGlobals Path"() -> (w615:path)
            n377 = call "convertOldSetlist_toCluster_v5.vi"("HW settings path"=w615, "Load pre 5.6 Globals?"=TRUE, "Procedure path"=w617, "Version Selection"=w612) -> ("Procedure Name"=w616:string, "Save Cluster"=w614:T14, "error out"=w613:errorcluster)  [unwired: 9 in]
            n378 = local write "Procedure Name"(w616) -> ()
            n379 = control-ref of="Select Layout"() -> (w622:refnum<vi>)
            n380 = call "LoadedCluster_toSetList_v5.vi"("Devices queue"=w606, "Layout Ref"=w622, "Save Cluster"=w614, "Table Ref in"=w607, "VariableManagerRef"=w608, "error in (no error)"=w613, "Defer Updates? (T)"=w621) -> ("Loaded Version"=w623:string, "DevNums"=w620:i32[], "Col array"=w619:refnum<class "Column.lvclass">[], "User defined functions"=w611:string)  [unwired: 3 in, 2 out]
            n381 = control-ref of="Old HWGlobals History"() -> (w625:refnum<vi>)
            n382 = local write "User defined functions"(w611) -> ()
            n383 = global write "NextMaster_v4.vi" "User Procedures"(w611) -> ()
            n384 = local write "Loaded Version"(w623) -> ()
            n385 = local write "DevNums"(w620) -> ()
            n386 = local write "Col array"(w619) -> ()
            n387 = call "Load_HistoryUpdate.vi"("History ref"=w625, "New Path"=w615) -> ()  [unwired: 1 in]
            n388 = property on="UpdateHWI Button" class="Bool (strict)"("DisabledEnum"=T10."Enabled" ("Disabled")) -> ()  [unwired: 2 in, 2 out]
          }
        }
        n389 = property on="Loading Text" class="Str"("Visible"=w604) -> ()  [unwired: 2 in, 2 out]
      }
      event "Old Procedure History": Value Change {
        n390 = event-data() -> ("NewVal"=w628:string)  [unwired: 1 in, 2 out]
        n391 = String To Path(string=w628) -> (path=w629:path)
        n392 = local write "Old Procedure Path"(w629) -> ()
      }
      event "Old HWGlobals History": Value Change {
        n393 = event-data() -> ("NewVal"=w630:string)  [unwired: 1 in, 2 out]
        n394 = String To Path(string=w630) -> (path=w631:path)
        n395 = local write "Old HWGlobals Path"(w631) -> ()
      }
      event "Debug: apply appearance": Value Change {
        n396 = event-data() -> ()  [unwired: 1 in, 3 out]
        n397 = local read "Devices queue"() -> (w632:refnum<queue>)
        n398 = local read "Col array"() -> (w641:refnum<class "Column.lvclass">[])
        n399 = call "ModeFromDevices.vi"("error in (no error)"=w635, "Devices queue"=w632) -> ("error out"=w634:errorcluster, "Mode Col"=w633:i32)  [unwired: 8 in]
        n400 = control-ref of="SetList Table"() -> (w640:refnum<vi>)
        n401 = local read "Defer Updates?"() -> (w637:bool)
        n402 = control-ref of="Select Layout"() -> (w638:refnum<vi>)
        n403 = call "ApplyTableAppearance_benchmarking.vi"("Defer Updates? (T)"=w637, "Layout Ring Ref"=w638, "error in (no error)"=w634, "Mode Index"=w633, "Col Array in"=w641, "Table Ref in"=w640) -> ("error out"=w636:errorcluster)  [unwired: 4 in, 1 out]
        n404 = invoke on="Debug: apply appearance" class="Bool (strict)" method="Reinit To Default"(error in=w636) -> (error out=w639:errorcluster)  [unwired: 2 in, 2 out]
      }
      event "UpdateHWI Button": Value Change {
        n405 = event-data() -> ("CtlRef"=w649:refnum<vi>)  [unwired: 1 in, 3 out]
        n406 = property class="Bool (strict)"(reference=w649, "Value"=FALSE) -> ()  [unwired: 1 in, 2 out]
        n407 = local read "Update Event"() -> (w645:refnum<user-event>)
        n408 = Bundle(0, TRUE) -> (w642:cluster{i32, bool})  [unwired: 1 in]
        n409 = property on="SequenceHistory" class="Tbl (strict)"("Value"=string[][] [["-1", "Waiting", ""]] ("SequenceHistory")) -> (error out=w647:errorcluster)  [unwired: 2 in, 1 out]
        n410 = Generate User Event(user event=w645, event data cluster=w642, error in=w647) -> ()  [unwired: 1 in, 2 out]
      }
      event User Event {
        # "VariableManager Update Events"
        n411 = event-data() -> ("UpdateEvent"=w650:string)  [unwired: 1 in, 4 out]
        n412 = case shown="\"SequenceIndices\", \"UpdateEvent\", \"Variables\", Default" w650 {
          frame "SequenceIndices", "UpdateEvent", "Variables", Default {
            # "Re-enable UpdateHWI button if there is a change to VariableManager definition"
            n413 = property on="UpdateHWI Button" class="Bool (strict)"("DisabledEnum"=T10."Enabled" ("Disabled")) -> ()  [unwired: 2 in, 2 out]
          }
          frame "VariableGroups" {
          }
          frame "SequenceValues" {
          }
          frame "LastAcquireValues" {
          }
          frame "StopUI" {
          }
        }
      }
      event "Run Seq Button": Value Change {
        n414 = event-data() -> ("CtlRef"=w653:refnum<vi>, "NewVal"=w654:bool)  [unwired: 1 in, 1 out]
        n415 = case shown="True" w654 {
          tunnel: w653 -> [_ w657]
          tunnel: [_ w656] -> w652
          frame False {
          }
          frame True {
            n416 = control-ref of="VariableManager"() -> (w659:refnum<vi>)
            n417 = call "GetTotalSequenceSteps.vi"("VariableManagerRef in"=w659) -> ("error out"=w658:errorcluster, "TotalSequenceSteps"=w655:i32)  [unwired: 8 in, 1 out]
            n418 = case shown="No Error" w658 {
              selector: w658 -> [_ w692]
              tunnel: w657 -> [_ w694]
              tunnel: [_ w692] -> w656
              tunnel: w655 -> [w666 _]
              frame No Error {
                w661 = T10."Disabled" ("Disabled")
                n419 = for {
                  N: w666 -> [_]
                  tunnel: [w687] -> w665 mode=indexing
                  i -> [w691]
                  n420 = Number To Decimal String(number=w691) -> (decimal integer string=w690:string)  [unwired: 1 in]
                  n421 = Build Array(w690, "Waiting", "") -> (w687:string[])
                }
                n422 = property on="Run Button" class="Bool (strict)"("DisabledEnum"=w661) -> ()  [unwired: 2 in, 2 out]
                n423 = property on="Run Seq Button" class="Bool (strict)"("DisabledEnum"=w661) -> ()  [unwired: 2 in, 2 out]
                n424 = property on="RandomSequence" class="Bool (strict)"("DisabledEnum"=w661) -> ("Value"=w660:bool)  [unwired: 2 in, 2 out]
                n425 = property on="StopExperiment" class="Bool (strict)"("DisabledEnum"=T10."Enabled" ("Disabled")) -> ()  [unwired: 2 in, 2 out]
                n426 = case shown="True" w660 {
                  tunnel: w666 -> [_ w674]
                  tunnel: w665 -> [w671 w673]
                  tunnel: [w671 w672] -> w664
                  frame False {
                  }
                  frame True {
                    n427 = for {
                      N: w674 -> [w685]
                      shift-right: [w682] -> _
                      shift-left: w673 -> [w683]
                      tunnel: [w678] -> w672 mode=indexing
                      i -> [w686]
                      n428 = Random Number (0-1)() -> (number: 0 to 1=w675:dbl)
                      n429 = Subtract(x=w685, y=w686) -> (x-y=w684:i32)
                      n430 = Multiply(x=w684, y=w675) -> (x*y=w677:dbl)
                      n431 = Round Toward -Infinity(1:w677) -> (0:w676:dbl)
                      n432 = Delete From Array(array=w683, length=1, index (row)=w676) -> (deleted portion=w680:string[][], array with subset deleted=w682:string[][])  [unwired: 1 in]
                      n433 = Index Array(array=w680, index (row)=0) -> (element=w678:string[])  [unwired: 1 in]
                    }
                  }
                }
                n434 = local read "Seq. Event"() -> (w668:refnum<user-event>)
                n435 = Bundle("milliseconds to wait"=u32 0, FALSE) -> (w669:cluster{"milliseconds to wait":u32, bool})  [unwired: 1 in]
                n436 = property on="SequenceHistory" class="Tbl (strict)"("Value"=w664) -> (error out=w663:errorcluster)  [unwired: 2 in, 1 out]
                n437 = Generate User Event(user event=w668, event data cluster=w669, error in=w663) -> ()  [unwired: 1 in, 2 out]
              }
              frame Error {
                n438 = property class="Bool (strict)"(reference=w694, "Value"=FALSE) -> ()  [unwired: 1 in, 2 out]
              }
            }
          }
        }
      }
      event "Run Button": Value Change {
        n439 = event-data() -> ("NewVal"=w695:bool)  [unwired: 1 in, 2 out]
        n440 = case shown="True" w695 {
          frame False {
          }
          frame True {
            w696 = T10."Disabled" ("Disabled")
            n441 = local read "Seq. Event"() -> (w702:refnum<user-event>)
            n442 = property on="SequenceHistory" class="Tbl (strict)"("Value"=string[][] [["-1", "Waiting", ""]] ("SequenceHistory")) -> (error out=w698:errorcluster)  [unwired: 2 in, 1 out]
            n443 = Bundle("dimension size"=0, FALSE) -> (w703:cluster{"dimension size":i32, bool})  [unwired: 1 in]
            n444 = Generate User Event(user event=w702, event data cluster=w703, error in=w698) -> ()  [unwired: 1 in, 2 out]
            n445 = property on="Run Button" class="Bool (strict)"("DisabledEnum"=w696) -> ()  [unwired: 2 in, 2 out]
            n446 = property on="Run Seq Button" class="Bool (strict)"("DisabledEnum"=w696) -> ()  [unwired: 2 in, 2 out]
            n447 = property on="RandomSequence" class="Bool (strict)"("DisabledEnum"=w696) -> ()  [unwired: 2 in, 2 out]
            n448 = property on="StopExperiment" class="Bool (strict)"("DisabledEnum"=T10."Enabled" ("Disabled")) -> ()  [unwired: 2 in, 2 out]
          }
        }
      }
      event "SequenceHistory": Mouse Down? {
        # "Mulligan functionality"
        n449 = event-data() -> ("CtlRef"=w708:refnum<vi>, "Coords"=w707:T13)  [unwired: 1 in, 3 out]
        n450 = invoke class="Tbl (strict)" method="Point To Row Column"(reference=w708, "Point"=w707) -> (reference out=w705:refnum<vi>, "InBounds"=w704:bool, "CellPosition"=w706:T5)  [unwired: 4 in, 3 out]
        n451 = case shown="True" w704 {
          tunnel: w706 -> [_ w715]
          tunnel: w705 -> [_ w714]
          frame False {
          }
          frame True {
            # "If click in table"
            n452 = property class="Tbl (strict)"(reference=w714) -> (reference out=w711:refnum<vi>, "Value"=w710:string[][])  [unwired: 1 in, 1 out]
            n453 = Unbundle(w715) -> ("Row"=w709:i32)  [unwired: 1 out]
            n454 = Index Array(array=w710, index (row)=w709, index (col)=1 ("disabled index (col)")) -> (element=w712:string)
            n455 = case shown="\"Waiting\"" w712 {
              tunnel: w711 -> [_ w717 w723]
              tunnel: w710 -> [_ w721 w727]
              tunnel: w709 -> [_ w720 w726]
              frame Default {
              }
              frame "Waiting" {
                n456 = Replace Array Subset(array=w721, new element="Complete", index (row)=w720, index (col)=1 ("disabled index (col)")) -> (w716:string[][])
                n457 = property class="Tbl (strict)"(reference=w717, "Value"=w716) -> ()  [unwired: 1 in, 2 out]
              }
              frame "Complete" {
                n458 = Replace Array Subset(array=w727, new element="Waiting", index (row)=w726, index (col)=1 ("disabled index (col)")) -> (w722:string[][])
                n459 = property class="Tbl (strict)"(reference=w723, "Value"=w722) -> ()  [unwired: 1 in, 2 out]
              }
            }
          }
        }
        n460 = event-data("Discard?"=w704) -> ()  [unwired: 4 in, 1 out]
      }
      event "Sequencing Error", "Update Error", "Table error": Value Change {
        n461 = event-data() -> ("NewVal"=w728:errorcluster)  [unwired: 1 in, 2 out]
        n462 = case shown="Error" w728 {
          frame No Error {
          }
          frame Error {
            # "If an error was generated in any part of the program, automatically open the Errors tab."
            n463 = property on="Tab Control" class="TabCtl (strict)"("Value"=T2."Errors" ("Tab Control")) -> ()  [unwired: 2 in, 2 out]
          }
        }
      }
    }
    "Table error" <- w45
    n464 = disable-structure shown="Enabled" {
      frame Enabled {
        # "diagnositc"
        n465 = local read "Table History"() -> (w50:T8)
        n466 = Unbundle By Name(w50) -> ("OldTable Array"=w49:T9)
        n467 = Array Size(array=w49) -> (size(s)=→"Hist. size":i32)
      }
      frame Disabled {
      }
    }
  }
  n468 = while {
    stop <- w730 stop-if-true
    # "Update Event Structure"
    n469 = local read "Dyn. Regist. Update Event"() -> (w731:refnum<event-registration>)
    n470 = event shown="[0] <Update Event>: User Event" {
      selector: w731 -> [_ _]
      dyn-events: _ -> [_ _]
      timeout: _ -> [_ _]
      tunnel: [_ w776] -> w730
      event User Event {
        n471 = event-data() -> ("Seq. Idx"=w732:i32, "Force?"=w733:bool)  [unwired: 1 in]
        n472 = case shown="True" w733 {
          tunnel: [_ w758] -> w734
          tunnel: w732 -> [_ w737]
          frame False {
          }
          frame True {
            # "prepend filenumber placeholder\n(overwritten in CycleX loop)"
            n473 = property on="SequenceHistory" class="Tbl (strict)"() -> ("Value"=w740:string[][])  [unwired: 2 in, 2 out]
            n474 = control-ref of="VariableManager"() -> (w753:refnum<vi>)
            n475 = Index Array(array=w740, index (row)=w737, index (col)=0 ("disabled index (col)")) -> (element=w741:string)
            n476 = Scan From String(format string="%d", input string=w741) -> (output 1=w736:i32)  [unwired: 3 in, 3 out]
            n477 = call "GetVariableValues.vi"("SequenceStep"=w736, "VariableManagerRef in"=w753) -> ("error out"=w750:errorcluster, "VariableValues"=w748:refnum<class "VariableValue.lvclass">[])  [unwired: 7 in, 1 out]
            n478 = control-ref of="SetList Table"() -> (w761:refnum<vi>)
            n479 = for {
              tunnel: w748 -> [w765] mode=indexing
              tunnel: [w766] -> w749 mode=indexing
              tunnel: [w764] -> w747 mode=indexing
              n480 = call "VariableValueToCluster.vi"("VariableValue"=w765) -> ("VariableValueCluster"=w764:cluster{"Name":string, "Value":dbl})  [unwired: 10 in]
              n481 = call "VariableValueToString.vi"("VariableValue"=w765) -> ("VariableValueString"=w766:string)  [unwired: 10 in]
            }
            n482 = Greater?(x=w736, y=-1) -> (0:w755:bool)
            n483 = property class="Tbl (strict)"(reference=w761, error in=w750) -> (error out=w751:errorcluster, "Value"=w757:string[][], "Column Headers[]"=w756:string[])  [unwired: 1 out]
            n484 = local read "Devices queue"() -> (w763:refnum<queue>)
            n485 = local read "DevNums"() -> (w762:i32[])
            n486 = Concatenate Strings(w749) -> (w745:string)
            n487 = call "SetList SWI to Devices.vi"("error in (no error)"=w751, "SWI table"=w757, "DevNums In"=w762, "Devices queue"=w763) -> ("error out"=w759:errorcluster, "Devices queue out"=w760:refnum<queue>)  [unwired: 5 in, 1 out]
            n488 = invoke on="SequenceHistory" class="Tbl (strict)" method="Set Cell Value"("X Index"=2 ("disabled index (col)"), "Y Index"=w737, "Value"=w745) -> ()  [unwired: 3 in, 6 out]
            n489 = call "SetList_ToString.vi"("Column Names"=w756, "Current  Variables"=w747, "Device Data"=w757) -> ("Igor Inform String"=w752:string)
            n490 = case shown="True" w755 {
              tunnel: w753 -> [w773 _]
              tunnel: w737 -> [w769 _]
              tunnel: w752 -> [w770 w775]
              tunnel: [w772 w774] -> w743
              frame True {
                n491 = call "Construct Sequence Variable Igor String.vi"("Current index"=w769, "VariableManagerRef"=w773) -> ("Igor Instruction String"=w771:string[])  [unwired: 9 in]
                n492 = Build Array (concatenate)(w771, w770) -> (w772:string[])
              }
              frame False {
                n493 = Build Array(w775) -> (w774:string[])
              }
            }
            n494 = call "Update HWI.vi"("Error In"=w759, "Current Variables"=w747, "Devices queue"=w760) -> ("Error Out"=w758:errorcluster)  [unwired: 2 in, 1 out]
            n495 = property on="Update Error" class="Clust (strict)"("Val(Sgnl)"=w758) -> ()  [unwired: 2 in, 2 out]
            n496 = case shown="..-1" w736 {
              tunnel: w758 -> [_ w767]
              frame 0, Default {
              }
              frame ..-1 {
                n497 = case shown="No Error" w767 {
                  frame No Error {
                    n498 = property on="UpdateHWI Button" class="Bool (strict)"("DisabledEnum"=T10."Disabled and Grayed Out" ("Disabled")) -> ()  [unwired: 2 in, 2 out]
                  }
                  frame Error {
                  }
                }
              }
            }
            n499 = Build Array (concatenate)("FileNumber=null\n", w743) -> (→"Igor Inform Array":string[])
          }
        }
        n500 = local read "Update Notifier"() -> (w735:refnum<notifier>)
        n501 = Send Notification(notification=w734, notifier=w735) -> ()  [unwired: 1 in, 2 out]
      }
      event "quit": Value Change {
        # "Tried adding local variable read of Quit outside event loop, but I think it wasn't being read properly.\nIs there a problem having three event loops checking quit? - CDH\nI think if you wanted it to work as intended with the read outside of the loop, you would need to set a timeout value and event case. - ZES"
        n502 = event-data() -> ("NewVal"=w776:bool)  [unwired: 1 in, 1 out]
      }
    }
  }
  n503 = property on="UpdateHWI Button" class="Bool (strict)"("DisabledEnum"=T10."Disabled and Grayed Out" ("Disabled")) -> ()  [unwired: 2 in, 2 out]
  n504 = property on="Loading Text" class="Str"("Visible"=FALSE ("Load from Disk")) -> ()  [unwired: 2 in, 2 out]
  n505 = case shown="False" "PreserveHist?" {
    frame False {
      w777 = T8 {"OldTable Array"=[], "Undo pointer"=0}  # Table History
      # "re-initialize to empty\nfor now"
      n506 = local write "Table History"(w777) -> ()
    }
    frame True {
    }
  }
  n507 = while {
    stop <- w778 stop-if-true
    # "Sequence Event Structure"
    n508 = local read "Dyn.\nRegist.\nSeq.\nEvent"() -> (w779:refnum<event-registration>)
    n509 = event shown="[0] <Seq Event>: User Event" {
      selector: w779 -> [_ _]
      dyn-events: _ -> [_ _]
      timeout: _ -> [_ _]
      tunnel: [_ w822] -> w778
      event User Event {
        n510 = event-data() -> ()  [unwired: 1 in, 2 out]
        n511 = property on="StopExperiment" class="Bool (strict)"() -> ("Value"=w780:bool)  [unwired: 2 in, 2 out]
        n512 = case shown="True" w780 {
          frame False {
            # "If running cycle, do not force update."
            # "Look for waiting sequence"
            # "Run Experiment"
            n513 = property on="SequenceHistory" class="Tbl (strict)"() -> ("Value"=w788:string[][])  [unwired: 2 in, 2 out]
            n514 = Index Array(array=w788, index (col)=1 ("disabled index (col)")) -> (element=w790:string[])  [unwired: 1 in]
            n515 = for {
              tunnel: w790 -> [w794] mode=indexing
              tunnel: [w792] -> w787
              tunnel: [w791] -> w785
              i -> [w791]
              stop <- w792 stop-if-true
              n516 = Equal?(x=w794, y="Waiting") -> (x = y?=w792:bool)
            }
            n517 = property on="SequenceHistory" class="Tbl (strict)"() -> ("Value"=w781:string[][])  [unwired: 2 in, 2 out]
            n518 = Index Array(array=w781, index (row)=w785, index (col)=0 ("disabled index (col)")) -> (element=w784:string)
            n519 = Not Equal?(x=w784, y="-1") -> (x != y?=w782:bool)
            n520 = case shown="True" w787 {
              tunnel: w785 -> [_ w799]
              tunnel: w782 -> [_ w798]
              frame False {
                w796 = T10."Enabled" ("Disabled")
                w797 = FALSE
                # "No waiting sequence"
                n521 = property on="Run Button" class="Bool (strict)"("Value"=w797, "DisabledEnum"=w796) -> ()  [unwired: 2 in, 2 out]
                n522 = property on="Run Seq Button" class="Bool (strict)"("Value"=w797, "DisabledEnum"=w796) -> ()  [unwired: 2 in, 2 out]
                n523 = property on="RandomSequence" class="Bool (strict)"("DisabledEnum"=w796) -> ()  [unwired: 2 in, 2 out]
                n524 = property on="StopExperiment" class="Bool (strict)"("Value"=w797, "DisabledEnum"=T10."Disabled and Grayed Out" ("Disabled")) -> ()  [unwired: 2 in, 2 out]
              }
              frame True {
                # "Run waiting  sequence"
                n525 = stacked-sequence {
                  seq-local: [_ w805 _ _] -> [_ _ _ w815]
                  tunnel: w799 -> [w801 w804 w812 w814]
                  tunnel: w798 -> [_ w803 _ _]
                  frame #0 {
                    # "Update SequenceHistory Status"
                    n526 = invoke on="SequenceHistory" class="Tbl (strict)" method="Set Cell Value"("X Index"=1 ("disabled index (col)"), "Y Index"=w801, "Value"="Programming") -> ()  [unwired: 3 in, 6 out]
                  }
                  frame #1 {
                    # "Row number of waiting sequence"
                    n527 = local read "Update Event"() -> (w810:refnum<user-event>)
                    n528 = local read "Update Notifier"() -> (w807:refnum<notifier>)
                    n529 = Bundle(w804, w803) -> (w809:cluster{i32, bool})  [unwired: 1 in]
                    n530 = Generate User Event(user event=w810, event data cluster=w809) -> (error out=w806:errorcluster)  [unwired: 2 in, 1 out]
                    n531 = Wait on Notification(notifier=w807, ignore previous (F)=TRUE, error in (no error)=w806) -> (notification=w805:errorcluster)  [unwired: 1 in, 3 out]
                  }
                  frame #2 {
                    # "Update SequenceHistory Status"
                    n532 = invoke on="SequenceHistory" class="Tbl (strict)" method="Set Cell Value"("X Index"=1 ("disabled index (col)"), "Y Index"=w812, "Value"="Executing") -> ()  [unwired: 3 in, 6 out]
                  }
                  frame #3 {
                    n533 = local read "CycleX Event"() -> (w817:refnum<user-event>)
                    n534 = Bundle(w814, FALSE) -> (w818:cluster{i32, bool})  [unwired: 1 in]
                    n535 = Generate User Event(user event=w817, event data cluster=w818, error in=w815) -> ()  [unwired: 1 in, 2 out]
                  }
                }
              }
            }
          }
          frame True {
            w820 = T10."Enabled" ("Disabled")
            w821 = FALSE
            # "Stop experiment when Stop request"
            n536 = property on="Run Button" class="Bool (strict)"("Value"=w821, "DisabledEnum"=w820) -> ()  [unwired: 2 in, 2 out]
            n537 = property on="Run Seq Button" class="Bool (strict)"("Value"=w821, "DisabledEnum"=w820) -> ()  [unwired: 2 in, 2 out]
            n538 = property on="RandomSequence" class="Bool (strict)"("DisabledEnum"=w820) -> ()  [unwired: 2 in, 2 out]
            n539 = property on="StopExperiment" class="Bool (strict)"("Value"=w821, "DisabledEnum"=T10."Disabled and Grayed Out" ("Disabled")) -> ()  [unwired: 2 in, 2 out]
          }
        }
      }
      event "quit": Value Change {
        n540 = event-data() -> ("NewVal"=w822:bool)  [unwired: 1 in, 1 out]
      }
    }
  }
  n541 = invoke on="quit" class="Bool (strict)" method="Reinit To Default"() -> ()  [unwired: 3 in, 3 out]
  n542 = while {
    i -> [w827]
    stop <- w823 stop-if-true
    # "Diagnostics..."
    n543 = flat-sequence {
      tunnel: [w836] -> w824
      frame #0 {
        n544 = Wait (ms)(milliseconds to wait=u32 100) -> ()  [unwired: 1 out]
      }
      frame #1 {
        n545 = property on="SetList Table" class="Tbl (strict)"() -> (error out=w832:errorcluster, "OwningVI"=w834:refnum<vi>)  [unwired: 2 in, 1 out]
        n546 = property on="SetList Table" class="Tbl (strict)"() -> ("Key Focus"=→"Key Focus":bool, "EditPos"=→"Edit Position":T5, "Selection Size"=→"Selection Size":T5, "Selection Start"=→"Selection Start":T5, "Index Values"=→"Index Values":T1)  [unwired: 2 in, 2 out]
        n547 = local read "quit"() -> (w836:bool)
        n548 = property class="VI"(reference=w834, error in=w832) -> (error out=w831:errorcluster, "Panel"=w833:refnum<vi>)  [unwired: 1 out]
        n549 = property class="Pnl"(reference=w833, error in=w831) -> ("DeferPanUpdts"=→"Defer Pnl Upd":bool)  [unwired: 2 out]
        n550 = local write "Val Change"(FALSE ("Val Change")) -> ()
      }
    }
    n551 = Not(x="Diag. loop?") -> (.not. x?=w825:bool)
    n552 = Or(x=w824, y=w825) -> (x .or. y?=w823:bool)
    "diag. loop cnt" <- w827
  }
  n553 = while {
    stop <- w841 stop-if-true
    # "Handles running CycleX, which runs once per step"
    n554 = local read "Dyn.\nRegist.\nCycleX\nEvent"() -> (w842:refnum<event-registration>)
    n555 = event shown="[0] <CycleX Event>: User Event" {
      selector: w842 -> [_ _]
      dyn-events: _ -> [_ _]
      timeout: _ -> [_ _]
      tunnel: [_ w879] -> w841
      event User Event {
        w857 = 0 ("index (row)")
        # "replace file number"
        # "If cycle run,\nwait again"
        n556 = event-data() -> ("Seq. Idx"=w854:i32)  [unwired: 1 in, 1 out]
        n557 = local read "File Number"() -> (w852:i32)
        n558 = local read "Igor Inform Array"() -> (w846:string[])
        n559 = property on="SequenceHistory" class="Tbl (strict)"() -> ("Value"=w863:string[][])  [unwired: 2 in, 2 out]
        n560 = Increment(x=w852) -> (x+1=w851:i32)
        n561 = Format Into String(format string="FileNumber=%d\n", w852) -> (resulting string=w845:string)  [unwired: 2 in, 1 out]
        n562 = Index Array(array=w863, index (row)=w857, index (col)=w857) -> (element=w862:string)
        n563 = local write "File Number"(w851) -> ()
        n564 = shared-variable ".\\VariableLibrary.lvlib\\FileNum"(w851) -> ()  [unwired: 1 in, 1 out]
        n565 = Equal?(x="-1", y=w862) -> (x = y?=w859:bool)
        n566 = Replace Array Subset(array=w846, new element=w845, index=0) -> (w843:string[])
        n567 = Concatenate Strings(w843) -> (w853:string)
        "Igor Inform String" <- w853
        n568 = Build Array(w853) -> (w848:string[])
        n569 = local read "Devices queue"() -> (w867:refnum<queue>)
        n570 = call "CycleX.vi"("Devices queue"=w867, "Program only changes"="Program only changes", "Program during MOT loading"="Program during MOT loading", "Igor Inform String"=w848, "Additional wait time (s)"="Additional wait time (s)") -> ("error out"=w847:errorcluster)  [unwired: 10 in]
        n571 = property on="Cycle" class="Bool (strict)"(error in=w847) -> ("Value"=w860:bool)  [unwired: 1 in, 2 out]
        n572 = And(x=w860, y=w859) -> (x .and. y?=w858:bool)
        n573 = case shown="False" w858 {
          tunnel: ["Complete" "Waiting"] -> w855
          frame False {
          }
          frame True {
          }
        }
        n574 = invoke on="SequenceHistory" class="Tbl (strict)" method="Set Cell Value"("X Index"=1 ("disabled index (col)"), "Y Index"=w854, "Value"=w855) -> (error out=w850:errorcluster)  [unwired: 3 in, 5 out]
        n575 = case shown="Error" w847 {
          selector: w847 -> [w872 w878]
          tunnel: w850 -> [_ _]
          frame No Error {
            n576 = local read "Seq. Event"() -> (w873:refnum<user-event>)
            n577 = Bundle("milliseconds to wait"=u32 0, FALSE) -> (w874:cluster{"milliseconds to wait":u32, bool})  [unwired: 1 in]
            n578 = Generate User Event(user event=w873, event data cluster=w874, error in=w872) -> ()  [unwired: 1 in, 2 out]
          }
          frame Error {
            w876 = T10."Enabled" ("Disabled")
            w875 = FALSE
            n579 = property on="Sequencing Error" class="Clust (strict)"("Val(Sgnl)"=w878) -> ()  [unwired: 2 in, 2 out]
            n580 = property on="Run Button" class="Bool (strict)"("Value"=w875, "DisabledEnum"=w876) -> ()  [unwired: 2 in, 2 out]
            n581 = property on="Run Seq Button" class="Bool (strict)"("Value"=w875, "DisabledEnum"=w876) -> ()  [unwired: 2 in, 2 out]
            n582 = property on="RandomSequence" class="Bool (strict)"("DisabledEnum"=w876) -> ()  [unwired: 2 in, 2 out]
            n583 = property on="StopExperiment" class="Bool (strict)"("Value"=w875, "DisabledEnum"=T10."Disabled and Grayed Out" ("Disabled")) -> ()  [unwired: 2 in, 2 out]
          }
        }
      }
      event "quit": Value Change {
        n584 = event-data() -> ("NewVal"=w879:bool)  [unwired: 1 in, 1 out]
      }
    }
  }
